vi "Autonomous Independent.vi"() -> ()   [LabVIEW 2016]
doc: "This VI is called when autonomous begins, and will automatically be terminated when autonomous ends. You can carry out timed or sensor driven robot movement independently without needing to return to the caller."
uses:
  <vilib>/Rock Robotics/WPI/ThirdParty/CanMotor/TalonSRX/WPI_CANTalonSRX_APIFeedbackSelect.ctl
  <vilib>/Rock Robotics/WPI/ThirdParty/CanMotor/TalonSRX/WPI_CANTalonSRX_Params.ctl
  <vilib>/Rock Robotics/WPI/ThirdParty/CanMotor/TalonSRX/WPI_CANTalonSRX_APIControlMode.ctl
  <vilib>/Rock Robotics/WPI/Utilities/WPI_GetSetVariantRefNum.vi
  <vilib>/Rock Robotics/Network Tables/NT Read String.vi
  <vilib>/Rock Robotics/Network Tables/NT Write Numeric Array.vi
  <vilib>/Rock Robotics/WPI/RobotDrive/WPI_RobotDriveArcadeDrive_Standard(NoSaturation).vi
  Robot Global Data.vi
panel:
  out "PLAY 2":dbl
  out "PLAY 1":dbl
  in  "stop":bool
  out "Distance":dbl
  out "Current":dbl
  out "CURRENT":dbl
  out "Distance 5":dbl
  out "Distance 4":dbl
  out "Distance 3":dbl
  out "RIGHT SIDE":dbl
  out "Encoder Position 4":dbl
  out "Encoder Position 3":dbl
  out "Encoder Position":dbl
  out "Encoder Position 2":dbl
  # "Be sure to right-click and choose Data Operations>>Make Current Value default if you want to save the array values with the VI"
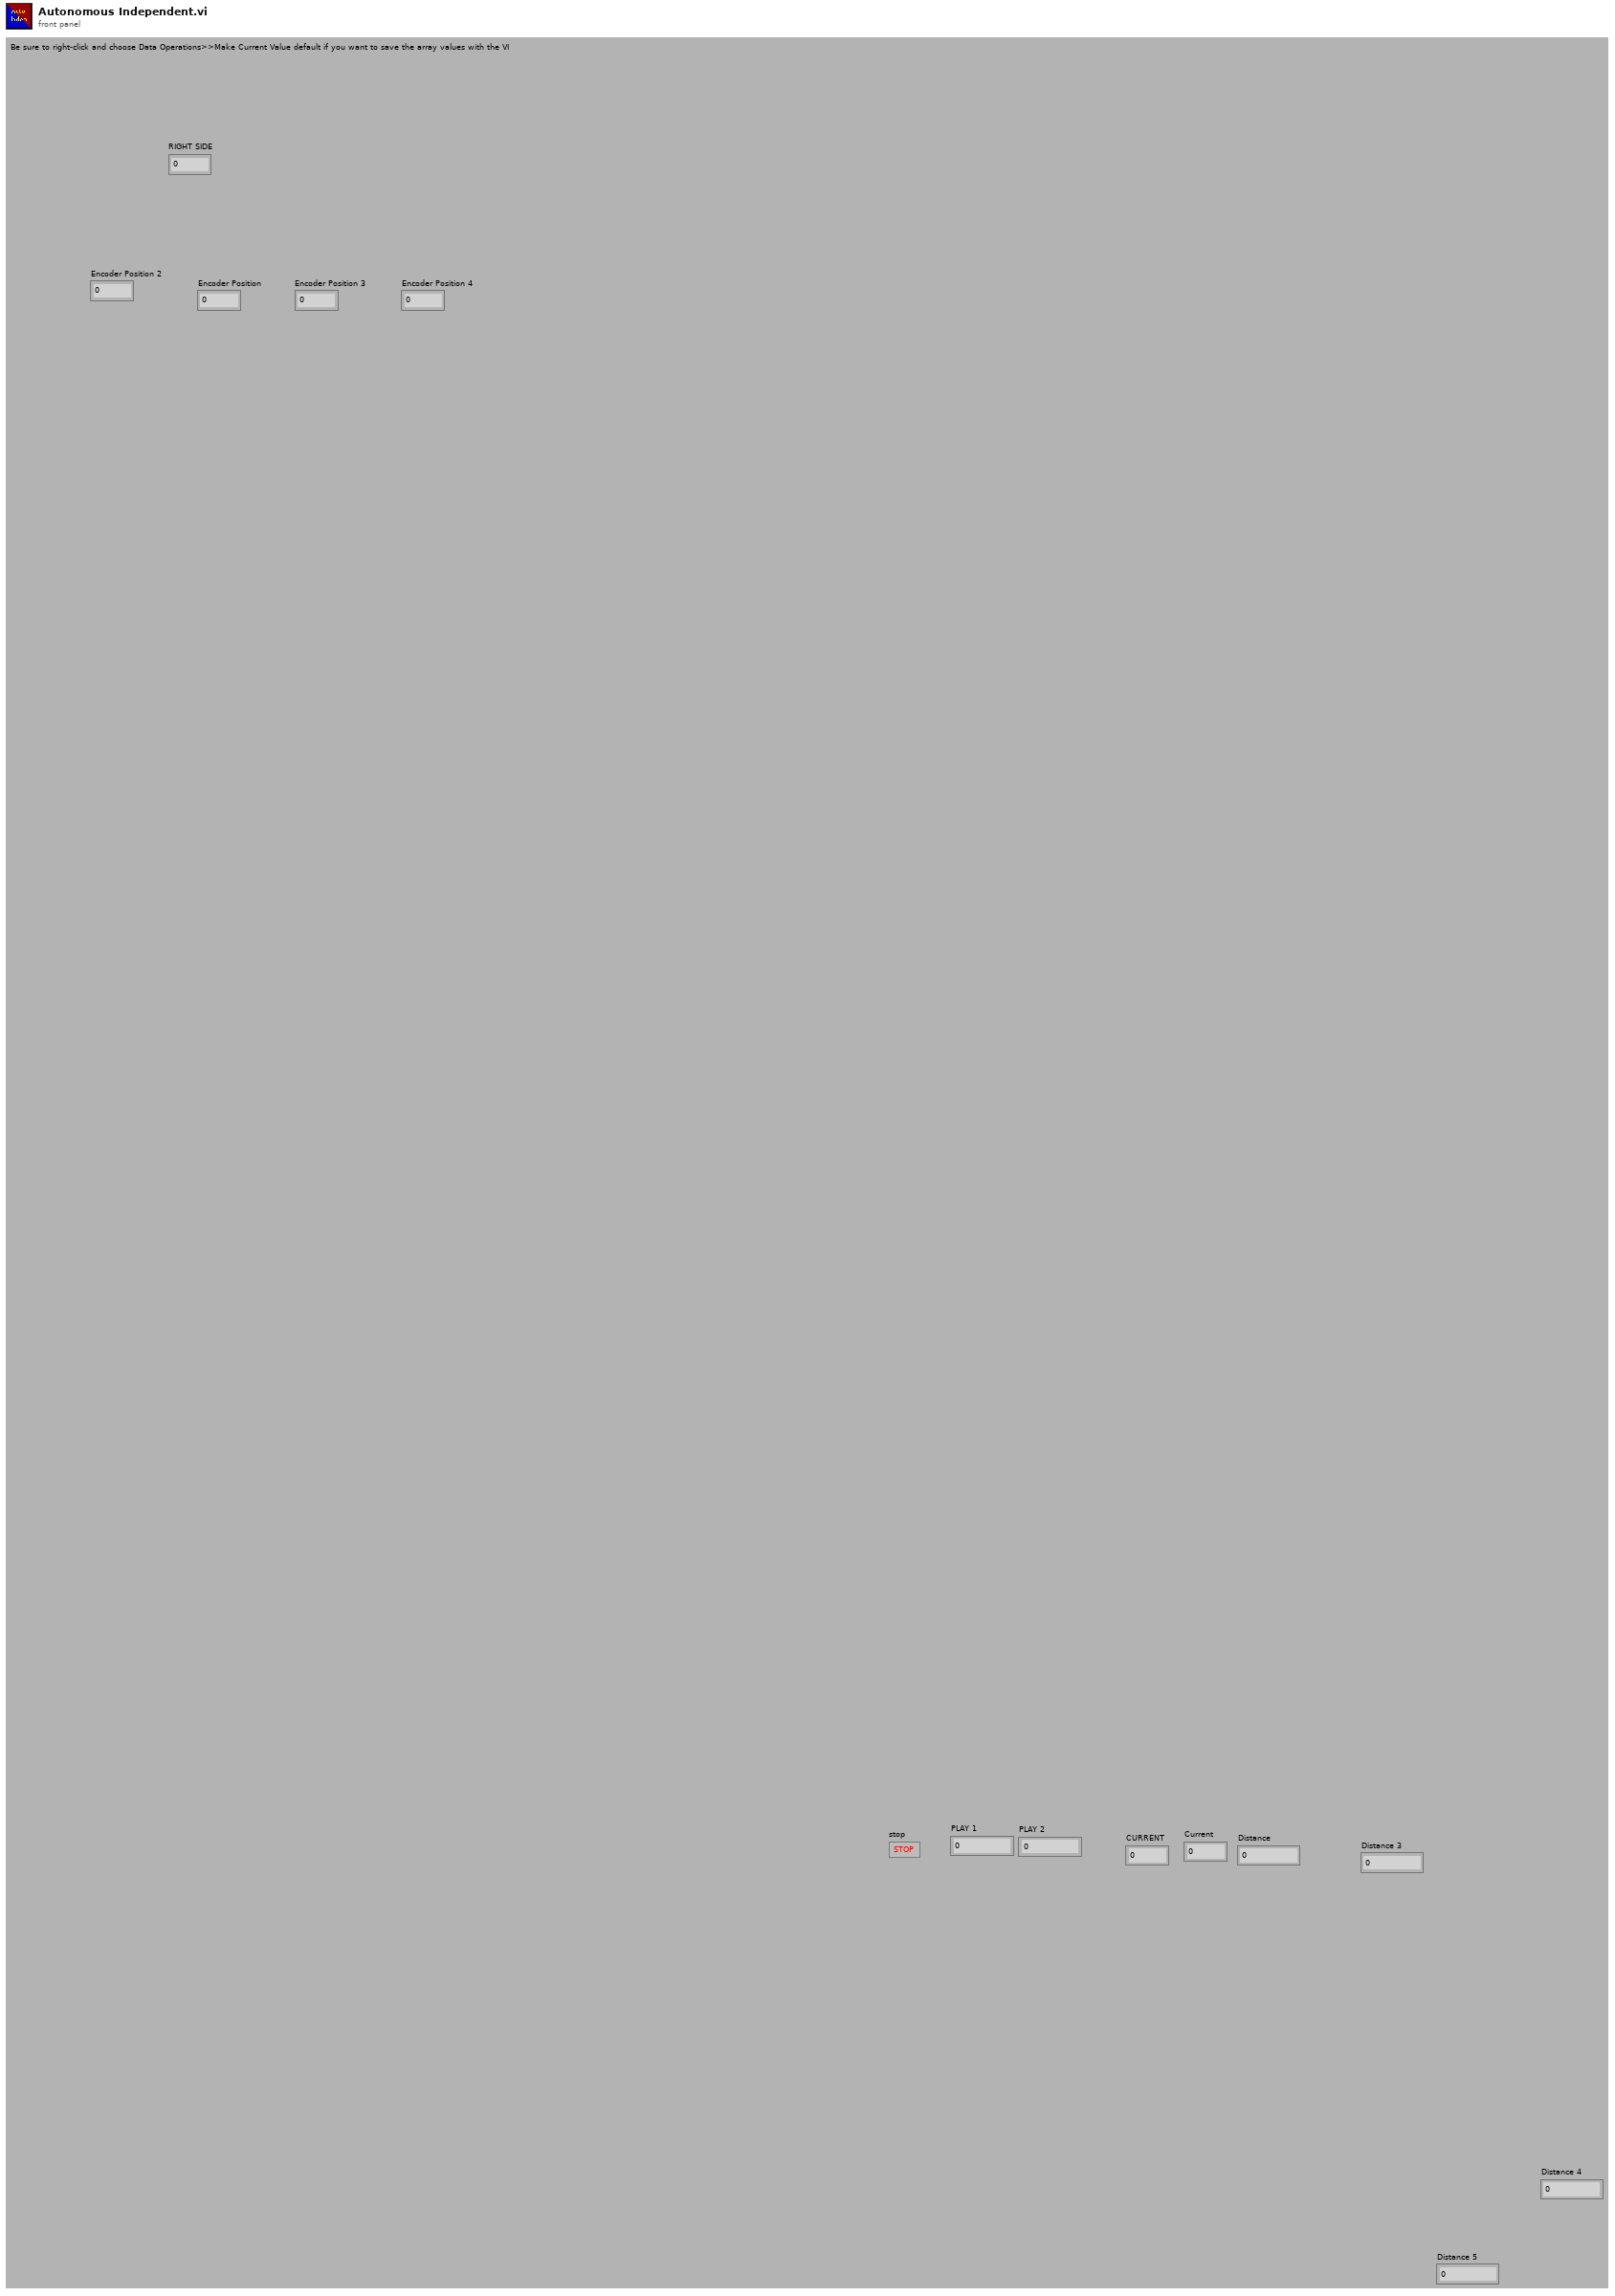
[diagram p1: front panel]
types:
  T1 = typedef "WPI_JoystickDevRef.ctl" = cluster{"Device":T2}
  T2 = typedef "WPI_JoystickDeviceEnum.ctl" = enum16{"USB 0", "USB 1", "USB 2", "USB 3", "USB 4", "USB 5"}
  T3 = typedef "WPI_EncoderDevRef.ctl" = cluster{"DevStatus":errorcluster, "EncoderIndex":T4, "CounterIndex":T5, "DistancePerCount":dbl, "Decoding Type":T6}
  T4 = typedef "FPGA_EncoderIdx.ctl" = enum8{"Enc 0", "Enc 1", "Enc 2", "Enc 3", "Enc 4", "Enc 5", "Enc 6", "Enc 7", "Invalid"}
  T5 = typedef "FPGA_CounterCtrSystemIndex.ctl" = enum8{"Ctr 0", "Ctr 1", "Ctr 2", "Ctr 3", "Ctr 4", "Ctr 5", "Ctr 6", "Ctr 7", "Invalid"}
  T6 = typedef "WPI_EncoderType.ctl" = enum16{"1x", "2x", "4x"}
  T7 = typedef "WPI_MotorControlDeviceRef.ctl" = cluster{"DeviceStatus":errorcluster, "Type":T8, "PWM":cluster{"PWM Channel":T9, "DeadBand":T10}, "CAN":cluster{"Device Number":u8, "SetOutput VI Ref":variant, "GetOutput VI Ref":variant, "Enable VI Ref":variant, "Disable VI Ref":variant, "Data":variant}, "Invert":bool}
  T8 = typedef "WPI_MotorControlType.ctl" = enum16{"PWM", "CAN"}
  T9 = typedef "FPGA_DIOPWMChannel.ctl" = enum8{"PWM 0", "PWM 1", "PWM 2", "PWM 3", "PWM 4", "PWM 5", "PWM 6", "PWM 7", "PWM 8", "PWM 9", "PWM MXP 0", "PWM MXP 1", "PWM MXP 2", "PWM MXP 3", "PWM MXP 4", "PWM MXP 5", "PWM MXP 6", "PWM MXP 7", "PWM MXP 8", "PWM MXP 9", "Invalid"}
  T10 = typedef "WPI_PWMDeadband.ctl" = cluster{"Name":string, "maxPositivePwm":i32, "minPositivePwm":i32, "centerPwm":i32, "maxNegativePwm":i32, "minNegativePwm":i32, "angularRange":u16}
  T11 = typedef "WPI_RobotDriveDevRef.ctl" = cluster{"DevStatus":errorcluster, "Motors[]":T7[], "Square Inputs":bool, "Max Output":dbl}
  T12 = typedef "WPI_CANTalonSRX_APIFeedbackSelect.ctl" = enum16{"Digital Quadrature Encoder", "Analog Potentiometer", "Analog Encoder", "Count on Quad-A (Rising-Edge)", "Count on Quad-A (Falling-Edge)", "CTR Magnetic Enc (Absolute)", "CTR Magnetic Enc (Relative)", "Pulse Width"}
  T13 = typedef "WPI_CANTalonSRX_APIControlMode.ctl" = enum8{"Percent VBus", "Speed", "Position", "Slave", "Unchanged / Invalid", "Voltage Compensation", "Current", "Motion Profile", "Motion Magic"}
  T14 = typedef "WPI_CANTalonSRX_Params.ctl" = u8
  T15 = typedef "WPI_CANTalonSRX_GlobalStatus.ctl" = cluster{"Applied Throttle":dbl, "Module Enabled":bool, "CAN Error":errorcluster, "Closed Loop Error":dbl, "Forward Limit Switch Closed":bool, "Reverse Limit Switch Closed":bool, "Sensor Position":dbl, "Sensor Velocity":dbl, "Current":dbl, "Sticky Fault - Over Temp":bool, "Sticky Fault - Under Voltage":bool, "Sticky Fault - Forward Limit":bool, "Sticky Fault - Reverse Limit":bool, "Sticky Fault - Forward Soft Limit":bool, "Sticky Fault - Reverse Soft Limit":bool, "Brake is Enabled":bool, "Encoder Position":dbl, "Encoder Velocity":dbl, "Encoder Index Count":dbl, "Encoder A Pin State":bool, "Encoder B Pin State":bool, "Encoder Index Pin State":bool, "Analog In":dbl, "Analog In Velocity":dbl, "Temperature (C)":dbl, "Battery Voltage":dbl, "Control 5 Is Supported":bool, "Current Profile Slot Select":dbl, "Pos Div 8":bool, "Vel Div 4":bool, "Pulse Width Position":i32, "Pulse Width Velocity":i32, "Pulse Width Rise To Rise (us)":i32, "Pulse Width Rise To Fall (us)":i32, "Mot Prof Active Is Under Run":bool, "Mot Prof Active Has Under Run":bool, "Mot Prof Active Is Last":bool, "Mot Prof Active Velocity Only":bool, "Mot Prof Active Is Valid":bool, "Mot Prof Buffer Is Full":bool, "Mot Prof Active Profile Slot Select":i32, "Mot Prof NextID":i32, "Mot Prof Count":i32, "Mot Prof Active Velocity":dbl, "Mot Prof Active Position":dbl, "Mot Prof Output Enable":i32, "UsageFrame":u32}
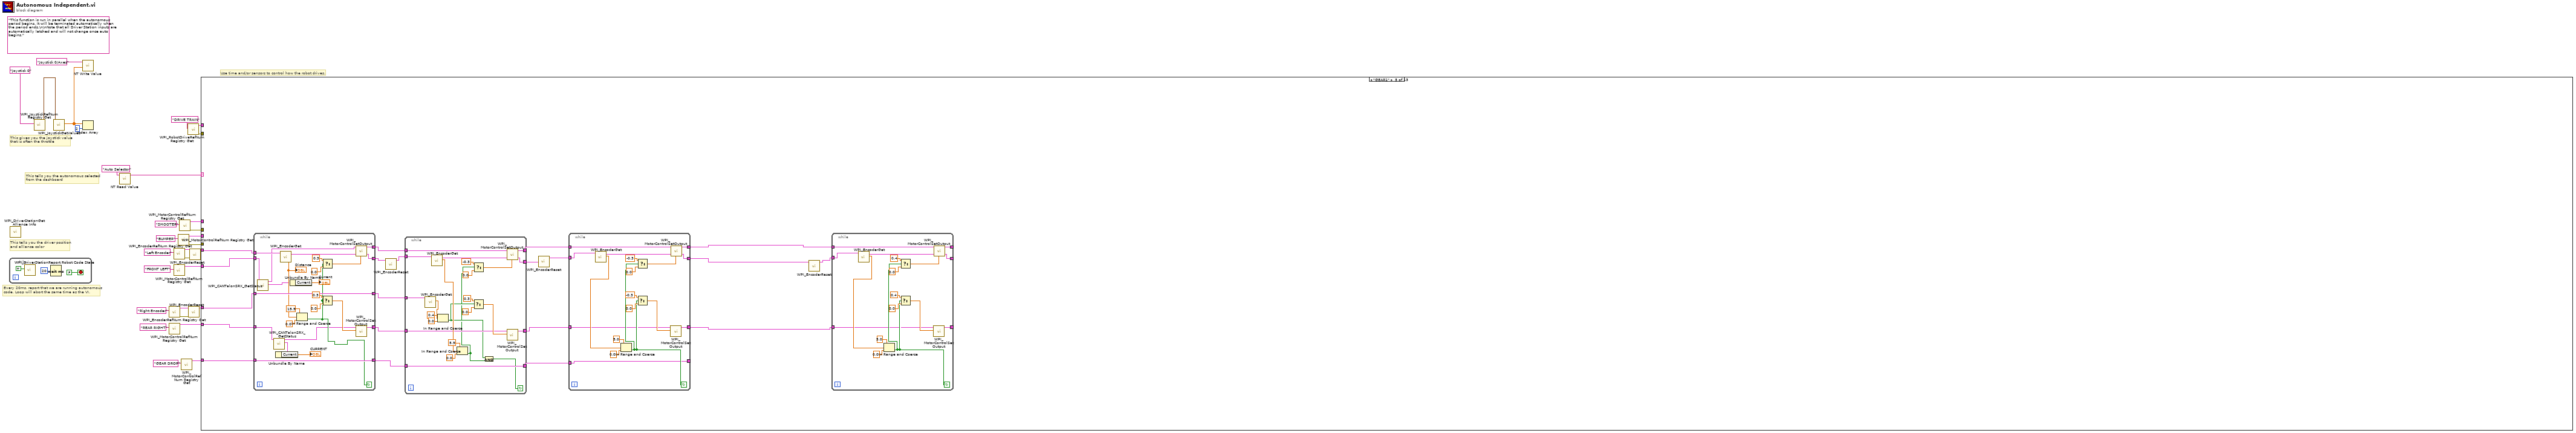
[diagram p0: block diagram]
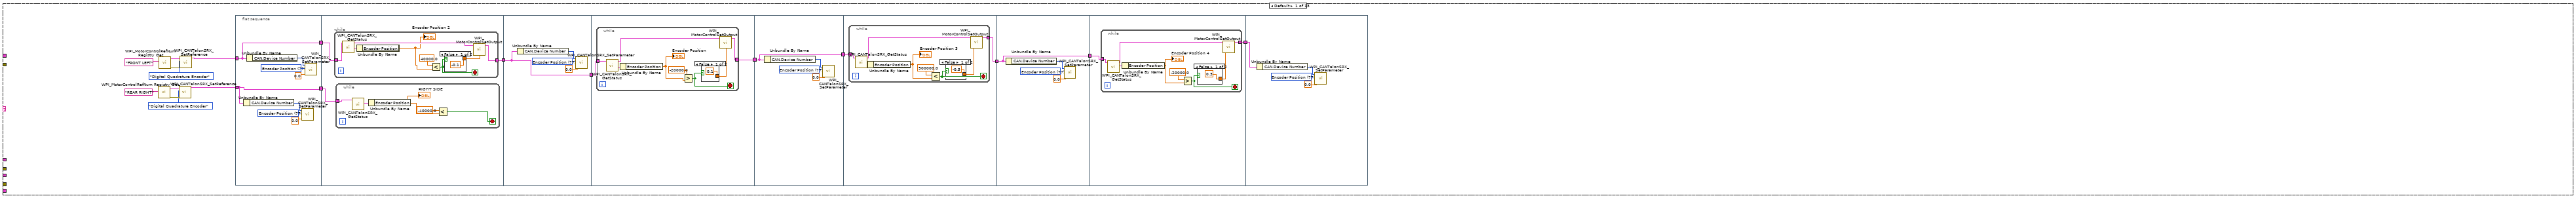
[diagram p2: hidden frame]
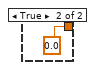
[diagram p3: hidden frame]
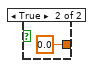
[diagram p4: hidden frame]
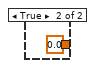
[diagram p5: hidden frame]
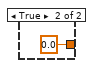
[diagram p6: hidden frame]
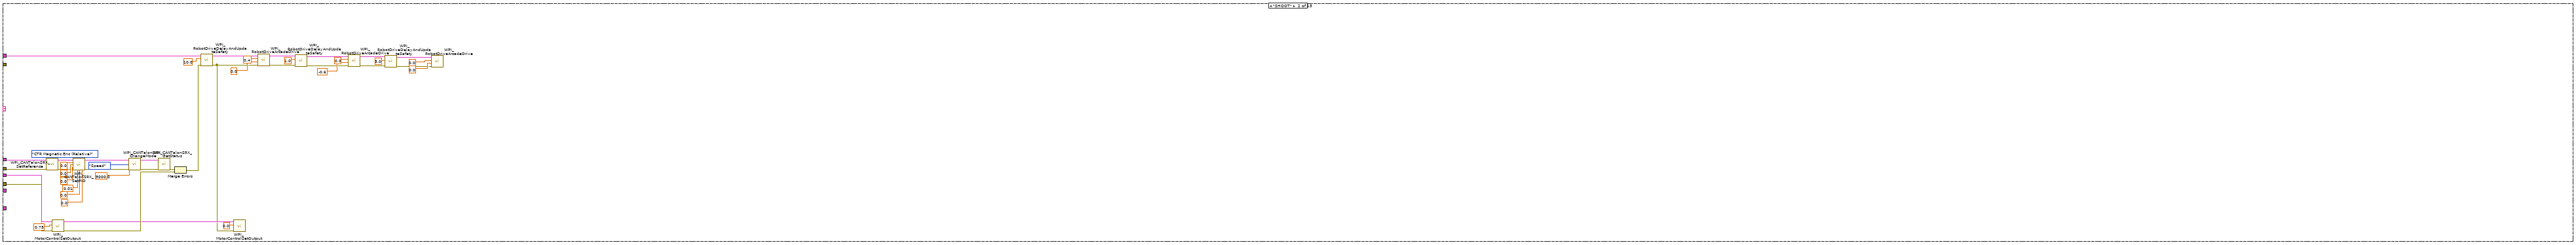
[diagram p7: hidden frame]
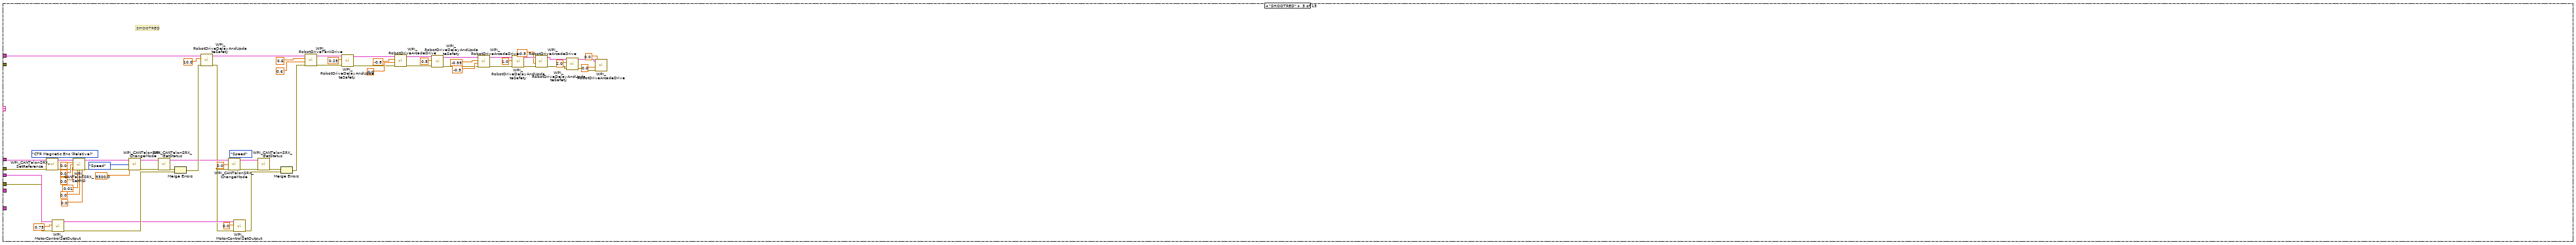
[diagram p8: hidden frame]
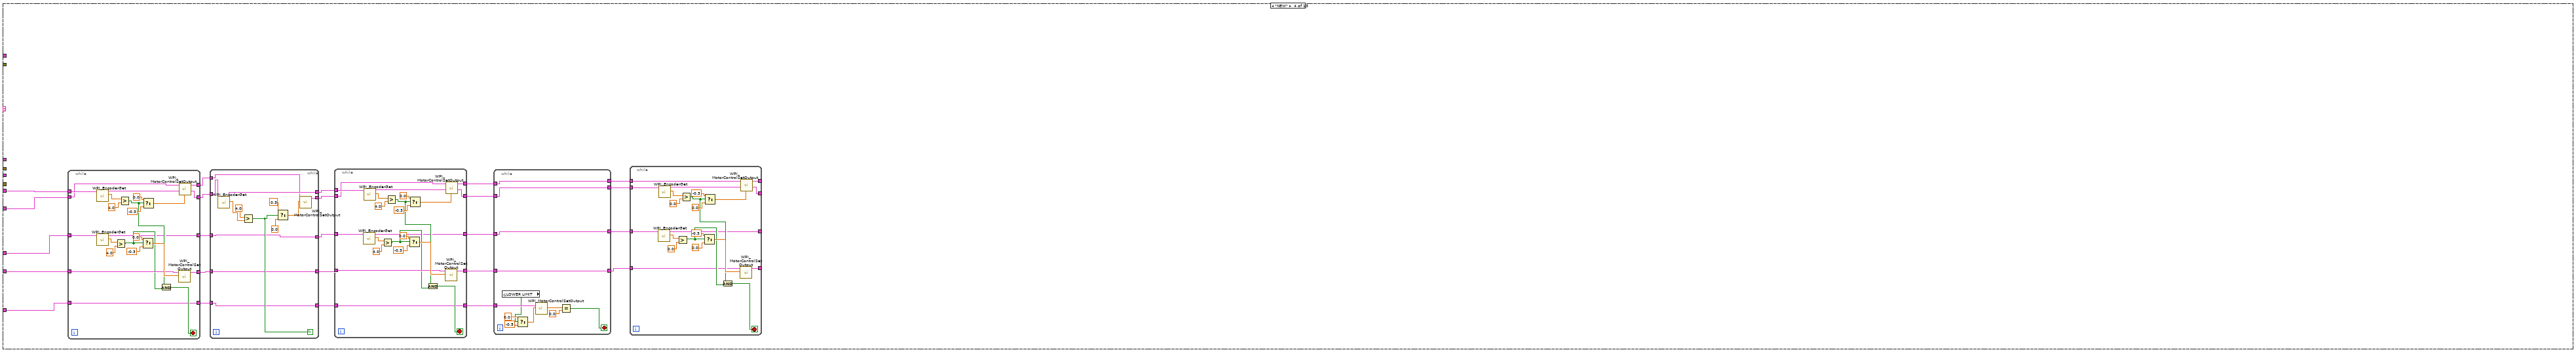
[diagram p9: hidden frame]
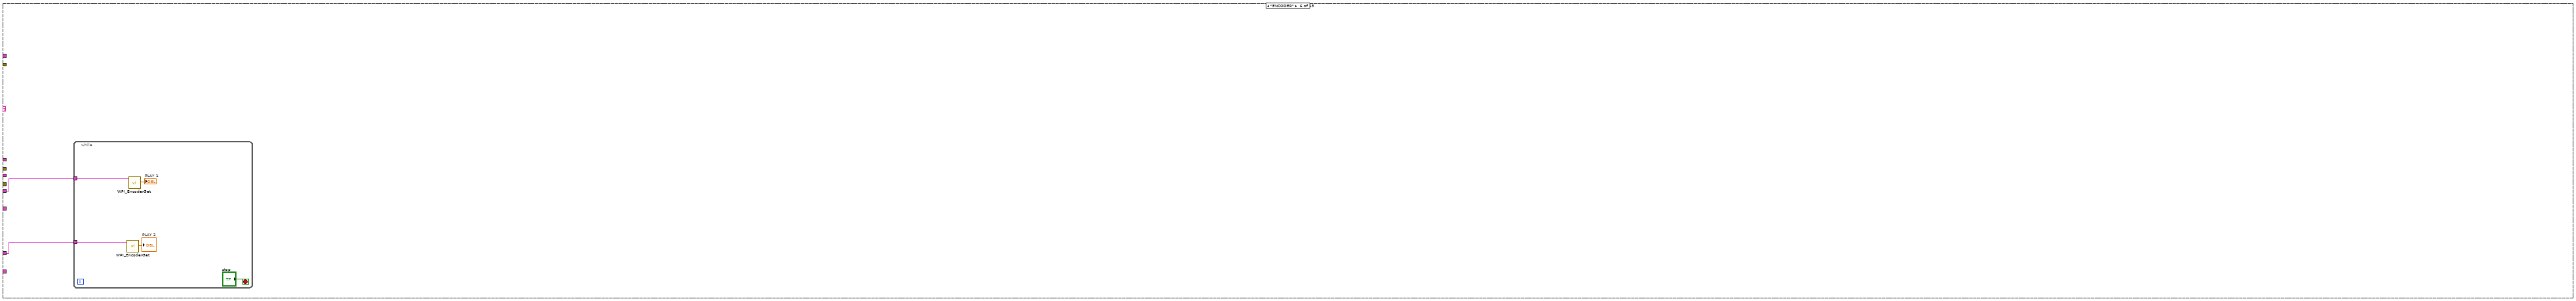
[diagram p10: hidden frame]
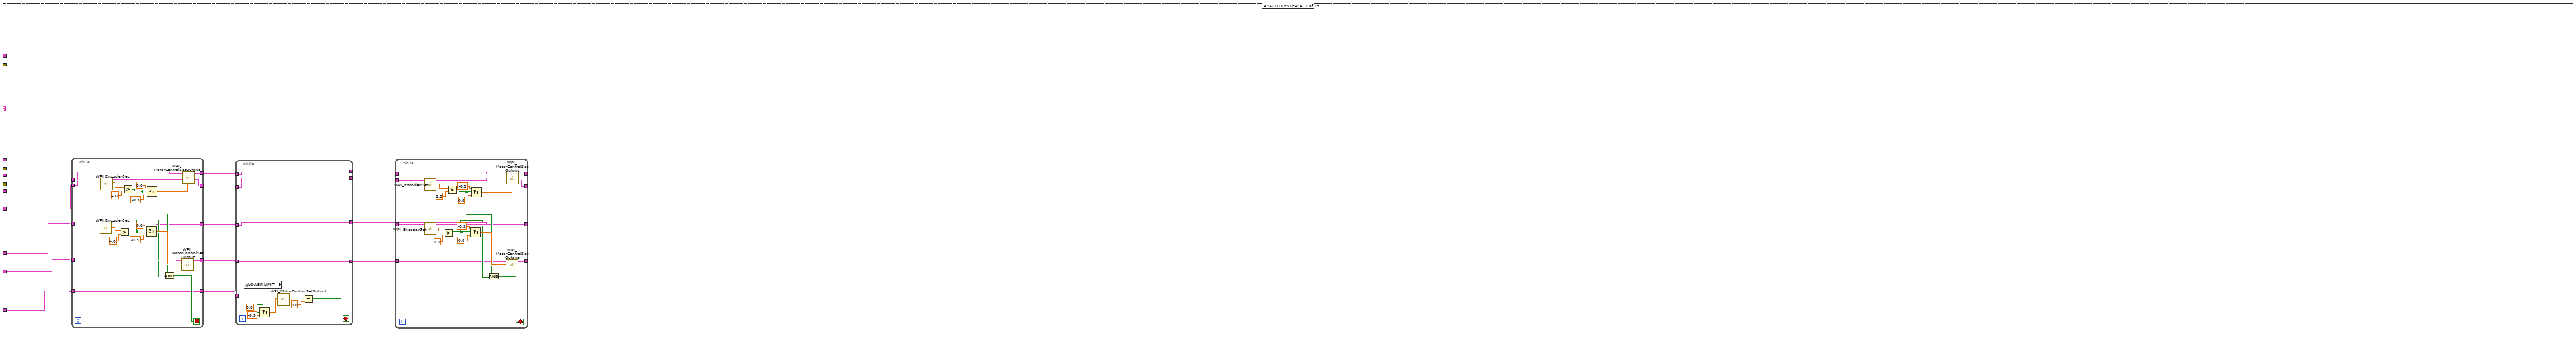
[diagram p11: hidden frame]
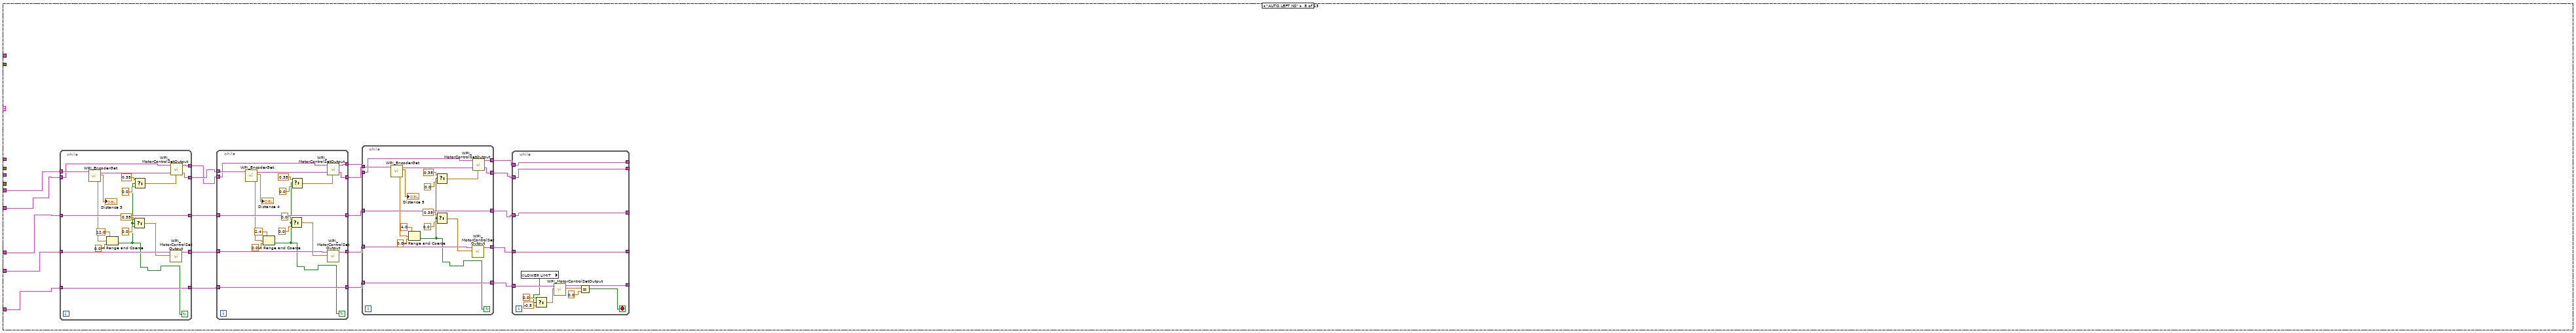
[diagram p12: hidden frame]
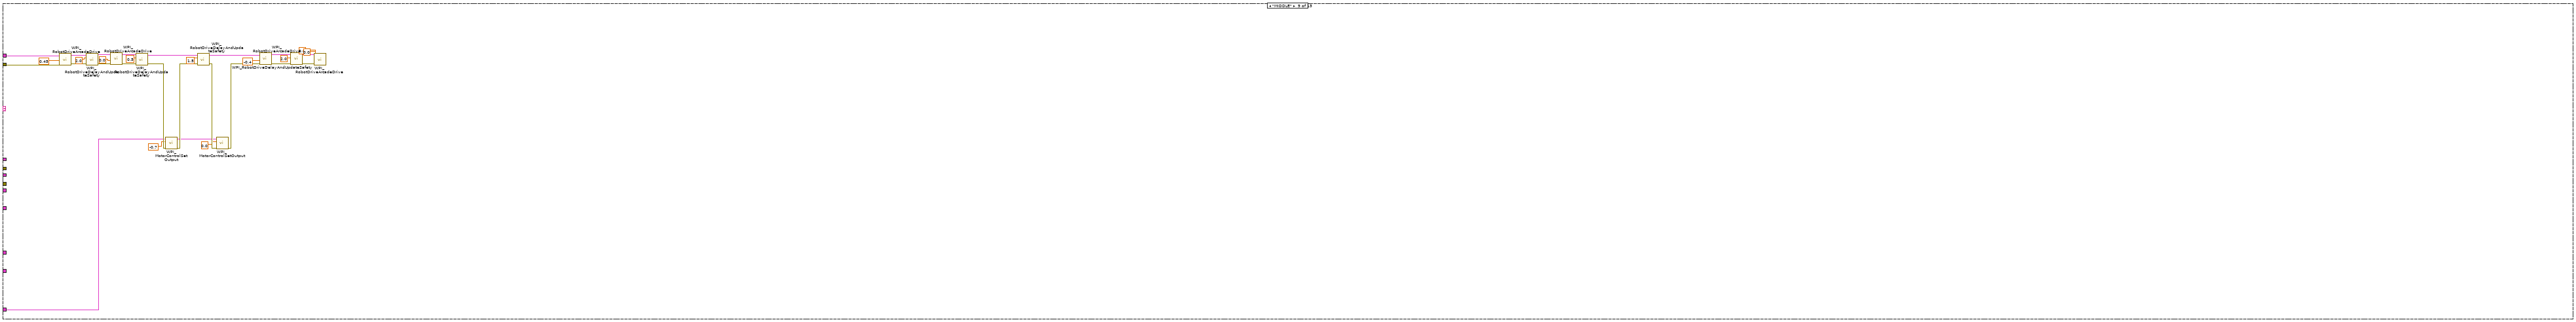
[diagram p13: hidden frame]
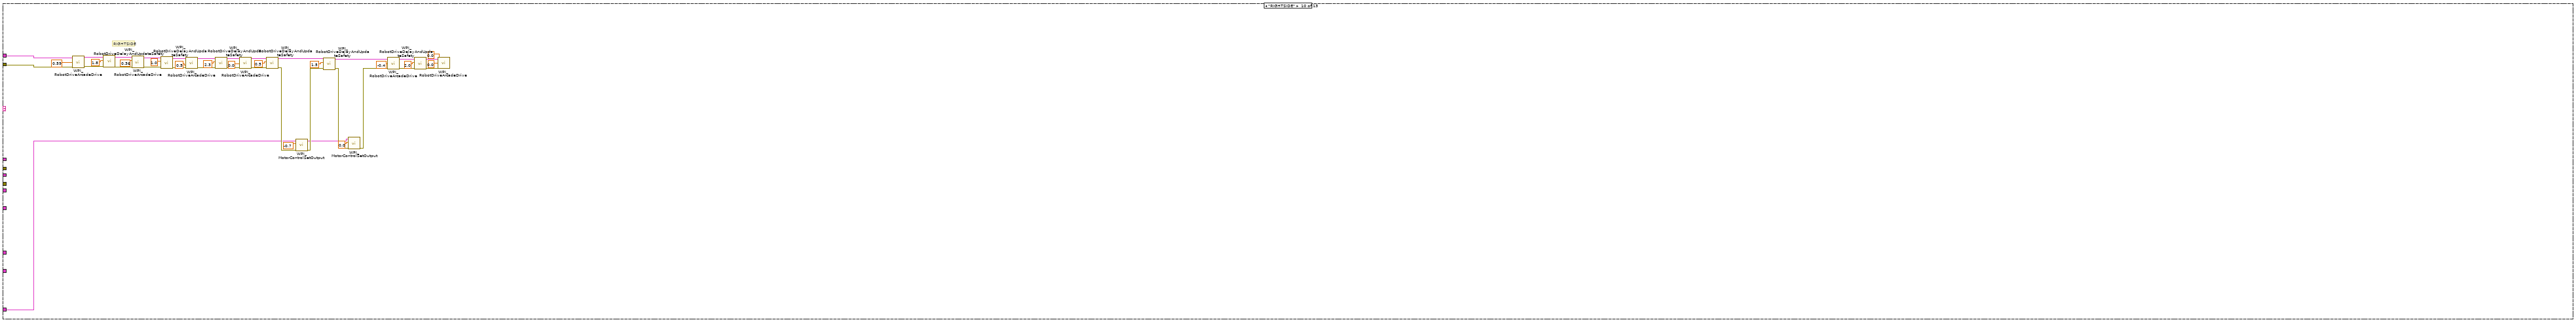
[diagram p14: hidden frame]
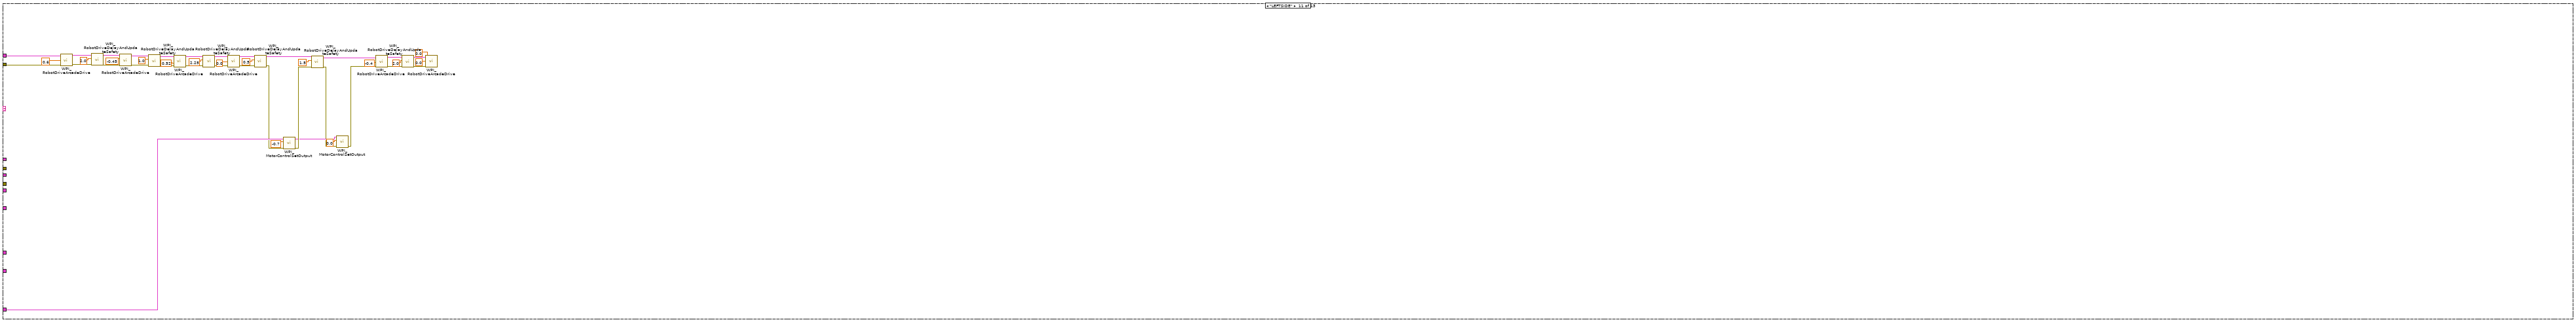
[diagram p15: hidden frame]
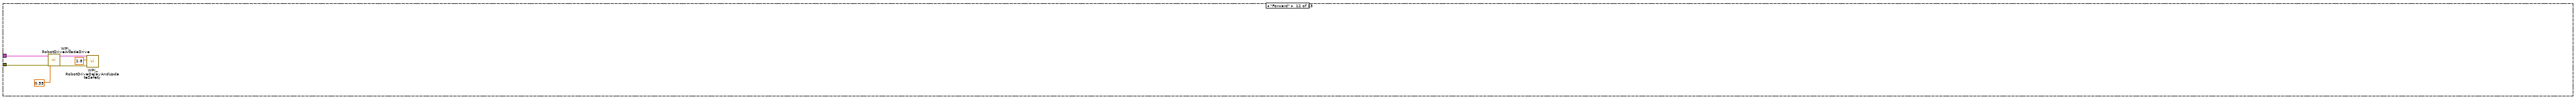
[diagram p16: hidden frame]
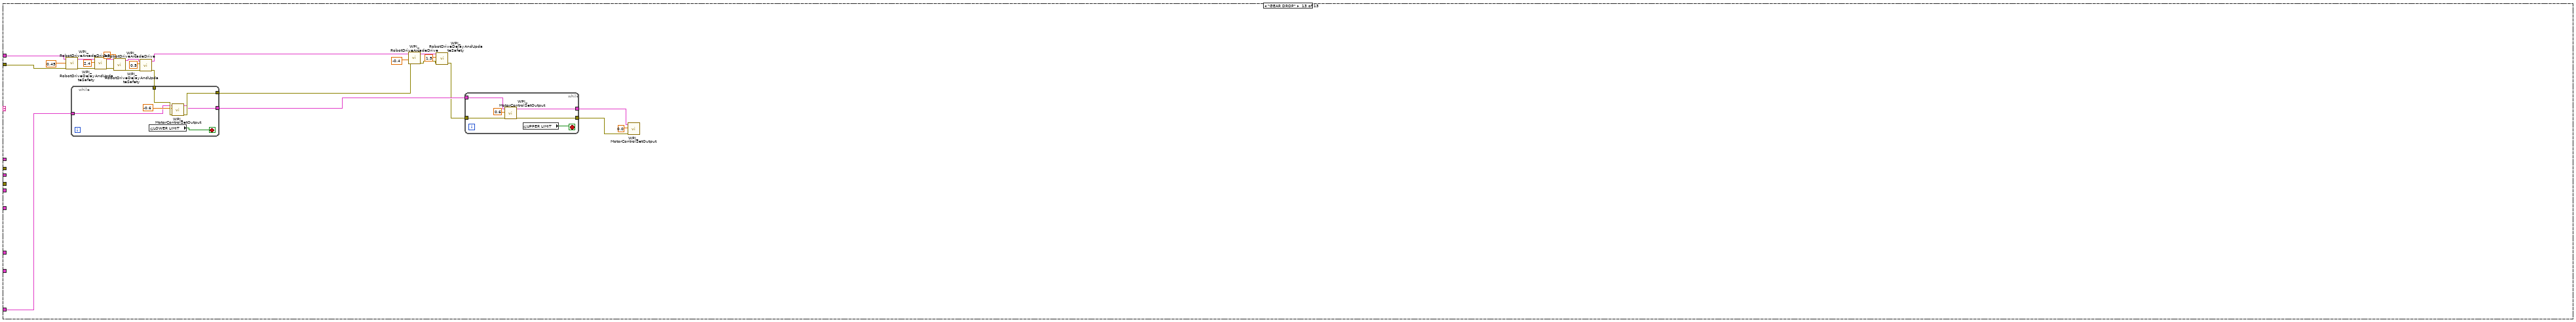
[diagram p17: hidden frame]
diagram:
  (unwired) "This function is run in parallel when the autonomous period begins. It will be terminated automatically when the period ends.\n\nNote that all Driver Station inputs are automatically latched and will not change once auto begins."
  # "Use time and/or sensors to control how the robot drives."
  # "This tells you the autonomous selected\nfrom the dashboard"
  # "Every 20ms, report that we are running autonomous\ncode. Loop will abort the same time as the VI."
  # "This gives you the joystick value\nthat is often the throttle"
  # "This tells you the driver position\nand alliance color"
  n1 = while {
    stop <- FALSE stop-if-true
    n2 = call <vilib>:"WPI_DriverStationReport Robot Code State.vi"("Autonomous"=TRUE) -> ()  [unwired: 10 in, 1 out]
    n3 = Wait (ms)(milliseconds to wait=u32 20) -> ()  [unwired: 1 out]
  }
  n4 = call <vilib>:"WPI_DriverStationGet Alliance Info.vi"() -> ()  [unwired: 12 out]
  n5 = call <vilib>:"WPI_JoystickRefNum Registry Get.vi"("refnum name"="Joystick 0") -> ("JoystickDevRef"=w29:T1)  [unwired: 1 in, 9 out]
  n6 = call <vilib>:"WPI_JoystickGetValues.vi"("JoystickDevRef"=w29) -> ("Axes"=w25:dbl[])  [unwired: 6 in, 4 out]
  n7 = call-poly <vilib>:"NT Write Value.vi"("Numeric Array"=w25, "Name"="Joystick 0/Axes") -> ()  [unwired: 9 in, 1 out]
  n8 = Index Array(array=w25, index=2) -> ()  [unwired: 1 out]
  n9 = call-poly <vilib>:"NT Read Value.vi"("Name"="Auto Selector") -> ("String"=w26:string)  [unwired: 9 in, 1 out]
  n10 = call <vilib>:"WPI_EncoderRefNum Registry Get.vi"("refnum name"="Right Encoder") -> ("error out"=w6:errorcluster, "EncoderDevRef"=w5:T3)  [unwired: 9 in]
  n11 = call <vilib>:"WPI_MotorControlRefNum Registry Get.vi"("refnum name"="REAR RIGHT") -> ("MotorControlDevRef"=w7:T7)  [unwired: 9 in, 1 out]
  n12 = call <vilib>:"WPI_EncoderRefNum Registry Get.vi"("refnum name"="Left Encoder") -> ("error out"=w3:errorcluster, "EncoderDevRef"=w2:T3)  [unwired: 9 in]
  n13 = call <vilib>:"WPI_MotorControlRefNum Registry Get.vi"("refnum name"="FRONT LEFT") -> ("MotorControlDevRef"=w10:T7)  [unwired: 9 in, 1 out]
  n14 = call <vilib>:"WPI_MotorControlRefNum Registry Get.vi"("refnum name"="BUMPER") -> ("error out"=w14:errorcluster, "MotorControlDevRef"=w15:T7)  [unwired: 9 in]
  n15 = call <vilib>:"WPI_MotorControlRefNum Registry Get.vi"("refnum name"="SHOOTER") -> ("error out"=w16:errorcluster, "MotorControlDevRef"=w17:T7)  [unwired: 9 in]
  n16 = call <vilib>:"WPI_MotorControlRefNum Registry Get.vi"("refnum name"="GEAR DROP") -> ("MotorControlDevRef"=w19:T7)  [unwired: 9 in, 1 out]
  n17 = call <vilib>:"WPI_RobotDriveRefNum Registry Get.vi"("refnum name"="DRIVE TRAIN") -> ("error out"=w21:errorcluster, "RobotDriveDevRef"=w22:T11)  [unwired: 9 in]
  n18 = call <vilib>:"WPI_EncoderReset.vi"("error in (no error)"=w6, "EncoderDevRef"=w5) -> ("EncoderDevRef"=w4:T3)  [unwired: 8 in, 1 out]
  n19 = call <vilib>:"WPI_EncoderReset.vi"("error in (no error)"=w3, "EncoderDevRef"=w2) -> ("EncoderDevRef"=w1:T3)  [unwired: 8 in, 1 out]
  n20 = case shown="\"GEAR1\"" w26 {
    tunnel: w22 -> [_ w157 w223 _ _ _ _ _ w649 w652 w735 w741 w766]
    tunnel: w21 -> [_ _ _ _ _ _ _ _ w648 w651 w734 w740 w765]
    tunnel: w19 -> [_ _ _ w249 w371 _ w472 w547 w636 w650 w711 _ w746]
    tunnel: w17 -> [_ w163 w229 _ _ _ _ _ _ _ _ _ _]
    tunnel: w16 -> [_ w162 w228 _ _ _ _ _ _ _ _ _ _]
    tunnel: w15 -> [_ w148 w216 _ _ _ _ _ _ _ _ _ _]
    tunnel: w14 -> [_ w147 w215 _ _ _ _ _ _ _ _ _ _]
    tunnel: w1 -> [_ _ _ w263 w374 w456 w476 w551 _ _ _ _ _]
    tunnel: w10 -> [_ _ _ w262 w375 _ w475 w550 _ _ _ _ _]
    tunnel: w7 -> [_ _ _ w260 w372 _ w473 w548 _ _ _ _ _]
    tunnel: w4 -> [_ _ _ w261 w373 w457 w474 w549 _ _ _ _ _]
    frame Default {
      n21 = call <vilib>:"WPI_MotorControlRefNum Registry Get.vi"("refnum name"="REAR RIGHT") -> ("error out"=w38:errorcluster, "MotorControlDevRef"=w37:T7)  [unwired: 9 in]
      n22 = call <vilib>:"WPI_MotorControlRefNum Registry Get.vi"("refnum name"="FRONT LEFT") -> ("error out"=w50:errorcluster, "MotorControlDevRef"=w51:T7)  [unwired: 9 in]
      n23 = call <vilib>:"WPI_CANTalonSRX_SetReference.vi"("error in (no error)"=w38, "Feedback Reference"=WPI_CANTalonSRX_APIFeedbackSelect."Digital Quadrature Encoder", "CAN Talon SRX Ref"=w37) -> ("CAN Talon SRX Ref"=w35:T7)  [unwired: 7 in, 1 out]
      n24 = call <vilib>:"WPI_CANTalonSRX_SetReference.vi"("error in (no error)"=w50, "Feedback Reference"=WPI_CANTalonSRX_APIFeedbackSelect."Digital Quadrature Encoder", "CAN Talon SRX Ref"=w51) -> ("CAN Talon SRX Ref"=w46:T7)  [unwired: 7 in, 1 out]
      n25 = flat-sequence {
        tunnel: w46 -> [w57]
        tunnel: [w57] -> w45
        tunnel: w35 -> [w53]
        tunnel: [w53] -> w34
        tunnel: [w62] -> w48
        tunnel: w45 -> [w63]
        tunnel: w34 -> [w61]
        tunnel: w48 -> [w79]
        tunnel: [w79] -> w47
        tunnel: w47 -> [w84]
        tunnel: [w83] -> w44
        tunnel: w44 -> [w95]
        tunnel: [w95] -> w43
        tunnel: w43 -> [w100]
        tunnel: [w99] -> w42
        tunnel: w42 -> [w111]
        tunnel: [w111] -> w41
        tunnel: w41 -> [w116]
        tunnel: [w115] -> w40
        tunnel: w40 -> [w127]
        frame #0 {
          w55 = T14 77 items=["Slot 0 - P"=1, "Slot 0 - I"=2, "Slot 0 - D"=3, "Slot 0 - F"=4, "Slot 0 - I Zone"=5, "Slot 0 - Ramp Rate"=6, "Slot 1 - P"=11, "Slot 1 - I"=12, "Slot 1 - D"=13, "Slot 1 - F"=14, "Slot 1 - I Zone"=15, "Slot 1 - Ramp Rate"=16, "Soft Limit - Forward"=21, "Soft Limit - Reverse"=22, "Soft Limit - Forward Enable"=23, "Soft Limit - Reverse Enable"=24, "On Boot - Brake Mode"=31, "On Boot - Limit Normally Closed - Forward"=32, "On Boot - Limit Normally Closed - Reverse"=33, "On Boot - Limit Disabled - Forward"=34, "On Boot - Limit Disabled - Reverse"=35, "Fault - Over Temp"=41, "Fault - Under Voltage"=42, "Fault - Forward Limit"=43, "Fault - Reverse Limit"=44, "Fault - Hardware Failure"=45, "Fault - Forward Soft Limit"=46, "Fault - Reverse Soft Limit"=47, "Sticky Fault - Over Temp"=48, "Sticky Fault - Under Voltage"=49, "Sticky Fault - Forward Limit"=50, "Sticky Fault - Reverse Limit"=51, "Sticky Fault - Forward Soft Limit"=52, "Sticky Fault - Reverse Soft Limit"=53, "Applied Throttle"=61, "Closed-Loop Error"=62, "Select Feedback Device"=63, "Reverse Closed-Loop Output"=64, "Mode Select"=65, "Profile Slot Select"=66, "Ramp Throttle"=67, "Reverse Feedback Sensor"=68, "Limit Switch Enabled"=69, "Limit Switch Closed - Forward"=70, "Limit Switch Closed - Reverse"=71, "Sensor Position"=73, "Sensor Velocity"=74, "Current"=75, "Brake is Enabled"=76, "Encoder Position"=77, "Encoder Velocity"=78, "Encoder Index Rise Events"=79, "Encoder A Pin State"=80, "Encoder B Pin State"=81, "Encoder Index Pin State"=82, "Analog In with Overflow"=83, "Analog In Velocity"=84, "Temperature"=85, "Battery Voltage"=86, "Reset Count"=87, "Reset Flags"=88, "Firmware Version"=89, "Settings Changed"=90, "Quad Filter Enable"=91, "Ignore Disable Broadcast"=92, "I Accumulator"=93, "Status 1 Frame Rate Ms"=94, "Status 2 Frame Rate Ms"=95, "Status 3 Frame Rate Ms"=96, "Status 4 Frame Rate Ms"=97, "Status 6 Frame Rate Ms"=98, "Status 7 Frame Rate Ms"=99, "Enable Index Pin Clear Position"=100, "Peak Positive Output"=104, "Nominal Positive Output"=105, "Peak Negative Output"=106, "Nominal Negative Output"=107, "Quad Index Pin Polarity"=108, "Status 8 Frame Rate Ms"=109, "Allow Position Overflow"=110, "Slot 0 - Allowable Closed-Loop Error"=111, "Number Potentiometer Turns"=112, "Encoder Codes Per Rev"=113, "Pulse Width Decoded Position"=114, "Analog Position"=115, "Voltage Compensation Rate (V/s)"=116, "Slot 1 - Allowable Closed-Loop Error"=117, "Motion Profile Has Underrun Err"=119, "Reserved 120"=120, "Legacy Control Mode"=121, "Motion Magic Acceleration"=122, "Motion Magic Cruise Velocity"=123, "Status 10 Frame Rate"=124, "Current Limit Threshold"=125, "CustomParam0"=137, "CustomParam1"=138, "PersStorageSaving"=139, "ClearPositionOnLimitF"=144, "ClearPositionOnLimitR"=145, "NominalBatteryVoltage"=146, "SampleVelocityPeriod"=147, "SampleVelocityWindow"=148] ("Parameter")
          w59 = T14 77 items=["Slot 0 - P"=1, "Slot 0 - I"=2, "Slot 0 - D"=3, "Slot 0 - F"=4, "Slot 0 - I Zone"=5, "Slot 0 - Ramp Rate"=6, "Slot 1 - P"=11, "Slot 1 - I"=12, "Slot 1 - D"=13, "Slot 1 - F"=14, "Slot 1 - I Zone"=15, "Slot 1 - Ramp Rate"=16, "Soft Limit - Forward"=21, "Soft Limit - Reverse"=22, "Soft Limit - Forward Enable"=23, "Soft Limit - Reverse Enable"=24, "On Boot - Brake Mode"=31, "On Boot - Limit Normally Closed - Forward"=32, "On Boot - Limit Normally Closed - Reverse"=33, "On Boot - Limit Disabled - Forward"=34, "On Boot - Limit Disabled - Reverse"=35, "Fault - Over Temp"=41, "Fault - Under Voltage"=42, "Fault - Forward Limit"=43, "Fault - Reverse Limit"=44, "Fault - Hardware Failure"=45, "Fault - Forward Soft Limit"=46, "Fault - Reverse Soft Limit"=47, "Sticky Fault - Over Temp"=48, "Sticky Fault - Under Voltage"=49, "Sticky Fault - Forward Limit"=50, "Sticky Fault - Reverse Limit"=51, "Sticky Fault - Forward Soft Limit"=52, "Sticky Fault - Reverse Soft Limit"=53, "Applied Throttle"=61, "Closed-Loop Error"=62, "Select Feedback Device"=63, "Reverse Closed-Loop Output"=64, "Mode Select"=65, "Profile Slot Select"=66, "Ramp Throttle"=67, "Reverse Feedback Sensor"=68, "Limit Switch Enabled"=69, "Limit Switch Closed - Forward"=70, "Limit Switch Closed - Reverse"=71, "Sensor Position"=73, "Sensor Velocity"=74, "Current"=75, "Brake is Enabled"=76, "Encoder Position"=77, "Encoder Velocity"=78, "Encoder Index Rise Events"=79, "Encoder A Pin State"=80, "Encoder B Pin State"=81, "Encoder Index Pin State"=82, "Analog In with Overflow"=83, "Analog In Velocity"=84, "Temperature"=85, "Battery Voltage"=86, "Reset Count"=87, "Reset Flags"=88, "Firmware Version"=89, "Settings Changed"=90, "Quad Filter Enable"=91, "Ignore Disable Broadcast"=92, "I Accumulator"=93, "Status 1 Frame Rate Ms"=94, "Status 2 Frame Rate Ms"=95, "Status 3 Frame Rate Ms"=96, "Status 4 Frame Rate Ms"=97, "Status 6 Frame Rate Ms"=98, "Status 7 Frame Rate Ms"=99, "Enable Index Pin Clear Position"=100, "Peak Positive Output"=104, "Nominal Positive Output"=105, "Peak Negative Output"=106, "Nominal Negative Output"=107, "Quad Index Pin Polarity"=108, "Status 8 Frame Rate Ms"=109, "Allow Position Overflow"=110, "Slot 0 - Allowable Closed-Loop Error"=111, "Number Potentiometer Turns"=112, "Encoder Codes Per Rev"=113, "Pulse Width Decoded Position"=114, "Analog Position"=115, "Voltage Compensation Rate (V/s)"=116, "Slot 1 - Allowable Closed-Loop Error"=117, "Motion Profile Has Underrun Err"=119, "Reserved 120"=120, "Legacy Control Mode"=121, "Motion Magic Acceleration"=122, "Motion Magic Cruise Velocity"=123, "Status 10 Frame Rate"=124, "Current Limit Threshold"=125, "CustomParam0"=137, "CustomParam1"=138, "PersStorageSaving"=139, "ClearPositionOnLimitF"=144, "ClearPositionOnLimitR"=145, "NominalBatteryVoltage"=146, "SampleVelocityPeriod"=147, "SampleVelocityWindow"=148] ("Parameter")
          n26 = Unbundle By Name(w53) -> ("CAN.Device Number"=w54:u8)
          n27 = Unbundle By Name(w57) -> ("CAN.Device Number"=w60:u8)
          n28 = call <vilib>:"WPI_CANTalonSRX_SetParameter.vi"("Value"=0.0, "Parameter"=w55, "Device ID (0)"=w54) -> ()  [unwired: 7 in, 2 out]
          n29 = call <vilib>:"WPI_CANTalonSRX_SetParameter.vi"("Value"=0.0, "Parameter"=w59, "Device ID (0)"=w60) -> ()  [unwired: 7 in, 2 out]
        }
        frame #1 {
          n30 = while {
            tunnel: w63 -> [w70]
            tunnel: [w69] -> w62
            stop <- w73 stop-if-true
            n31 = call <vilib>:"WPI_CANTalonSRX_GetStatus.vi"("CAN Talon SRX Ref"=w70) -> ("Talon SRX Status"=w76:T15, "CAN Talon SRX Ref"=w75:T7)  [unwired: 8 in, 1 out]
            n32 = Unbundle By Name(w76) -> ("Encoder Position"=w72:dbl)
            "Encoder Position 2" <- w72
            n33 = Less?(x=40000.0, y=w72) -> (x < y?=w73:bool)
            n34 = case shown="False" w73 {
              tunnel: [-0.1 ("x") 0.0 ("x")] -> w74
              frame False {
              }
              frame True {
              }
            }
            n35 = call <vilib>:"WPI_MotorControlSetOutput.vi"("Output"=w74, "MotorControlDevRef"=w75) -> ("MotorControlDevRef"=w69:T7)  [unwired: 7 in, 2 out]
          }
          n36 = while {
            tunnel: w61 -> [w68]
            stop <- w65 stop-if-true
            n37 = call <vilib>:"WPI_CANTalonSRX_GetStatus.vi"("CAN Talon SRX Ref"=w68) -> ("Talon SRX Status"=w64:T15)  [unwired: 8 in, 2 out]
            n38 = Unbundle By Name(w64) -> ("Encoder Position"=w67:dbl)
            "RIGHT SIDE" <- w67
            n39 = Less?(x=-40000.0, y=w67) -> (x < y?=w65:bool)
          }
        }
        frame #2 {
          w81 = T14 77 items=["Slot 0 - P"=1, "Slot 0 - I"=2, "Slot 0 - D"=3, "Slot 0 - F"=4, "Slot 0 - I Zone"=5, "Slot 0 - Ramp Rate"=6, "Slot 1 - P"=11, "Slot 1 - I"=12, "Slot 1 - D"=13, "Slot 1 - F"=14, "Slot 1 - I Zone"=15, "Slot 1 - Ramp Rate"=16, "Soft Limit - Forward"=21, "Soft Limit - Reverse"=22, "Soft Limit - Forward Enable"=23, "Soft Limit - Reverse Enable"=24, "On Boot - Brake Mode"=31, "On Boot - Limit Normally Closed - Forward"=32, "On Boot - Limit Normally Closed - Reverse"=33, "On Boot - Limit Disabled - Forward"=34, "On Boot - Limit Disabled - Reverse"=35, "Fault - Over Temp"=41, "Fault - Under Voltage"=42, "Fault - Forward Limit"=43, "Fault - Reverse Limit"=44, "Fault - Hardware Failure"=45, "Fault - Forward Soft Limit"=46, "Fault - Reverse Soft Limit"=47, "Sticky Fault - Over Temp"=48, "Sticky Fault - Under Voltage"=49, "Sticky Fault - Forward Limit"=50, "Sticky Fault - Reverse Limit"=51, "Sticky Fault - Forward Soft Limit"=52, "Sticky Fault - Reverse Soft Limit"=53, "Applied Throttle"=61, "Closed-Loop Error"=62, "Select Feedback Device"=63, "Reverse Closed-Loop Output"=64, "Mode Select"=65, "Profile Slot Select"=66, "Ramp Throttle"=67, "Reverse Feedback Sensor"=68, "Limit Switch Enabled"=69, "Limit Switch Closed - Forward"=70, "Limit Switch Closed - Reverse"=71, "Sensor Position"=73, "Sensor Velocity"=74, "Current"=75, "Brake is Enabled"=76, "Encoder Position"=77, "Encoder Velocity"=78, "Encoder Index Rise Events"=79, "Encoder A Pin State"=80, "Encoder B Pin State"=81, "Encoder Index Pin State"=82, "Analog In with Overflow"=83, "Analog In Velocity"=84, "Temperature"=85, "Battery Voltage"=86, "Reset Count"=87, "Reset Flags"=88, "Firmware Version"=89, "Settings Changed"=90, "Quad Filter Enable"=91, "Ignore Disable Broadcast"=92, "I Accumulator"=93, "Status 1 Frame Rate Ms"=94, "Status 2 Frame Rate Ms"=95, "Status 3 Frame Rate Ms"=96, "Status 4 Frame Rate Ms"=97, "Status 6 Frame Rate Ms"=98, "Status 7 Frame Rate Ms"=99, "Enable Index Pin Clear Position"=100, "Peak Positive Output"=104, "Nominal Positive Output"=105, "Peak Negative Output"=106, "Nominal Negative Output"=107, "Quad Index Pin Polarity"=108, "Status 8 Frame Rate Ms"=109, "Allow Position Overflow"=110, "Slot 0 - Allowable Closed-Loop Error"=111, "Number Potentiometer Turns"=112, "Encoder Codes Per Rev"=113, "Pulse Width Decoded Position"=114, "Analog Position"=115, "Voltage Compensation Rate (V/s)"=116, "Slot 1 - Allowable Closed-Loop Error"=117, "Motion Profile Has Underrun Err"=119, "Reserved 120"=120, "Legacy Control Mode"=121, "Motion Magic Acceleration"=122, "Motion Magic Cruise Velocity"=123, "Status 10 Frame Rate"=124, "Current Limit Threshold"=125, "CustomParam0"=137, "CustomParam1"=138, "PersStorageSaving"=139, "ClearPositionOnLimitF"=144, "ClearPositionOnLimitR"=145, "NominalBatteryVoltage"=146, "SampleVelocityPeriod"=147, "SampleVelocityWindow"=148] ("Parameter")
          n40 = Unbundle By Name(w79) -> ("CAN.Device Number"=w82:u8)
          n41 = call <vilib>:"WPI_CANTalonSRX_SetParameter.vi"("Value"=0.0, "Parameter"=w81, "Device ID (0)"=w82) -> ()  [unwired: 7 in, 2 out]
        }
        frame #3 {
          n42 = while {
            tunnel: w84 -> [w86]
            tunnel: [w85] -> w83
            stop <- w89 stop-if-true
            n43 = call <vilib>:"WPI_CANTalonSRX_GetStatus.vi"("CAN Talon SRX Ref"=w86) -> ("Talon SRX Status"=w92:T15, "CAN Talon SRX Ref"=w91:T7)  [unwired: 8 in, 1 out]
            n44 = Unbundle By Name(w92) -> ("Encoder Position"=w88:dbl)
            "Encoder Position" <- w88
            n45 = Greater?(x=-20000.0 ("y"), y=w88) -> (0:w89:bool)
            n46 = case shown="False" w89 {
              tunnel: [0.1 ("x") 0.0 ("x")] -> w90
              frame False {
              }
              frame True {
              }
            }
            n47 = call <vilib>:"WPI_MotorControlSetOutput.vi"("Output"=w90, "MotorControlDevRef"=w91) -> ("MotorControlDevRef"=w85:T7)  [unwired: 7 in, 2 out]
          }
        }
        frame #4 {
          w97 = T14 77 items=["Slot 0 - P"=1, "Slot 0 - I"=2, "Slot 0 - D"=3, "Slot 0 - F"=4, "Slot 0 - I Zone"=5, "Slot 0 - Ramp Rate"=6, "Slot 1 - P"=11, "Slot 1 - I"=12, "Slot 1 - D"=13, "Slot 1 - F"=14, "Slot 1 - I Zone"=15, "Slot 1 - Ramp Rate"=16, "Soft Limit - Forward"=21, "Soft Limit - Reverse"=22, "Soft Limit - Forward Enable"=23, "Soft Limit - Reverse Enable"=24, "On Boot - Brake Mode"=31, "On Boot - Limit Normally Closed - Forward"=32, "On Boot - Limit Normally Closed - Reverse"=33, "On Boot - Limit Disabled - Forward"=34, "On Boot - Limit Disabled - Reverse"=35, "Fault - Over Temp"=41, "Fault - Under Voltage"=42, "Fault - Forward Limit"=43, "Fault - Reverse Limit"=44, "Fault - Hardware Failure"=45, "Fault - Forward Soft Limit"=46, "Fault - Reverse Soft Limit"=47, "Sticky Fault - Over Temp"=48, "Sticky Fault - Under Voltage"=49, "Sticky Fault - Forward Limit"=50, "Sticky Fault - Reverse Limit"=51, "Sticky Fault - Forward Soft Limit"=52, "Sticky Fault - Reverse Soft Limit"=53, "Applied Throttle"=61, "Closed-Loop Error"=62, "Select Feedback Device"=63, "Reverse Closed-Loop Output"=64, "Mode Select"=65, "Profile Slot Select"=66, "Ramp Throttle"=67, "Reverse Feedback Sensor"=68, "Limit Switch Enabled"=69, "Limit Switch Closed - Forward"=70, "Limit Switch Closed - Reverse"=71, "Sensor Position"=73, "Sensor Velocity"=74, "Current"=75, "Brake is Enabled"=76, "Encoder Position"=77, "Encoder Velocity"=78, "Encoder Index Rise Events"=79, "Encoder A Pin State"=80, "Encoder B Pin State"=81, "Encoder Index Pin State"=82, "Analog In with Overflow"=83, "Analog In Velocity"=84, "Temperature"=85, "Battery Voltage"=86, "Reset Count"=87, "Reset Flags"=88, "Firmware Version"=89, "Settings Changed"=90, "Quad Filter Enable"=91, "Ignore Disable Broadcast"=92, "I Accumulator"=93, "Status 1 Frame Rate Ms"=94, "Status 2 Frame Rate Ms"=95, "Status 3 Frame Rate Ms"=96, "Status 4 Frame Rate Ms"=97, "Status 6 Frame Rate Ms"=98, "Status 7 Frame Rate Ms"=99, "Enable Index Pin Clear Position"=100, "Peak Positive Output"=104, "Nominal Positive Output"=105, "Peak Negative Output"=106, "Nominal Negative Output"=107, "Quad Index Pin Polarity"=108, "Status 8 Frame Rate Ms"=109, "Allow Position Overflow"=110, "Slot 0 - Allowable Closed-Loop Error"=111, "Number Potentiometer Turns"=112, "Encoder Codes Per Rev"=113, "Pulse Width Decoded Position"=114, "Analog Position"=115, "Voltage Compensation Rate (V/s)"=116, "Slot 1 - Allowable Closed-Loop Error"=117, "Motion Profile Has Underrun Err"=119, "Reserved 120"=120, "Legacy Control Mode"=121, "Motion Magic Acceleration"=122, "Motion Magic Cruise Velocity"=123, "Status 10 Frame Rate"=124, "Current Limit Threshold"=125, "CustomParam0"=137, "CustomParam1"=138, "PersStorageSaving"=139, "ClearPositionOnLimitF"=144, "ClearPositionOnLimitR"=145, "NominalBatteryVoltage"=146, "SampleVelocityPeriod"=147, "SampleVelocityWindow"=148] ("Parameter")
          n48 = Unbundle By Name(w95) -> ("CAN.Device Number"=w98:u8)
          n49 = call <vilib>:"WPI_CANTalonSRX_SetParameter.vi"("Value"=0.0, "Parameter"=w97, "Device ID (0)"=w98) -> ()  [unwired: 7 in, 2 out]
        }
        frame #5 {
          n50 = while {
            tunnel: w100 -> [w102]
            tunnel: [w101] -> w99
            stop <- w105 stop-if-true
            n51 = call <vilib>:"WPI_CANTalonSRX_GetStatus.vi"("CAN Talon SRX Ref"=w102) -> ("Talon SRX Status"=w108:T15, "CAN Talon SRX Ref"=w107:T7)  [unwired: 8 in, 1 out]
            n52 = Unbundle By Name(w108) -> ("Encoder Position"=w104:dbl)
            "Encoder Position 3" <- w104
            n53 = Less?(x=500000.0, y=w104) -> (x < y?=w105:bool)
            n54 = case shown="False" w105 {
              tunnel: [-0.5 ("x") 0.0 ("x")] -> w106
              frame False {
              }
              frame True {
              }
            }
            n55 = call <vilib>:"WPI_MotorControlSetOutput.vi"("Output"=w106, "MotorControlDevRef"=w107) -> ("MotorControlDevRef"=w101:T7)  [unwired: 7 in, 2 out]
          }
        }
        frame #6 {
          w113 = T14 77 items=["Slot 0 - P"=1, "Slot 0 - I"=2, "Slot 0 - D"=3, "Slot 0 - F"=4, "Slot 0 - I Zone"=5, "Slot 0 - Ramp Rate"=6, "Slot 1 - P"=11, "Slot 1 - I"=12, "Slot 1 - D"=13, "Slot 1 - F"=14, "Slot 1 - I Zone"=15, "Slot 1 - Ramp Rate"=16, "Soft Limit - Forward"=21, "Soft Limit - Reverse"=22, "Soft Limit - Forward Enable"=23, "Soft Limit - Reverse Enable"=24, "On Boot - Brake Mode"=31, "On Boot - Limit Normally Closed - Forward"=32, "On Boot - Limit Normally Closed - Reverse"=33, "On Boot - Limit Disabled - Forward"=34, "On Boot - Limit Disabled - Reverse"=35, "Fault - Over Temp"=41, "Fault - Under Voltage"=42, "Fault - Forward Limit"=43, "Fault - Reverse Limit"=44, "Fault - Hardware Failure"=45, "Fault - Forward Soft Limit"=46, "Fault - Reverse Soft Limit"=47, "Sticky Fault - Over Temp"=48, "Sticky Fault - Under Voltage"=49, "Sticky Fault - Forward Limit"=50, "Sticky Fault - Reverse Limit"=51, "Sticky Fault - Forward Soft Limit"=52, "Sticky Fault - Reverse Soft Limit"=53, "Applied Throttle"=61, "Closed-Loop Error"=62, "Select Feedback Device"=63, "Reverse Closed-Loop Output"=64, "Mode Select"=65, "Profile Slot Select"=66, "Ramp Throttle"=67, "Reverse Feedback Sensor"=68, "Limit Switch Enabled"=69, "Limit Switch Closed - Forward"=70, "Limit Switch Closed - Reverse"=71, "Sensor Position"=73, "Sensor Velocity"=74, "Current"=75, "Brake is Enabled"=76, "Encoder Position"=77, "Encoder Velocity"=78, "Encoder Index Rise Events"=79, "Encoder A Pin State"=80, "Encoder B Pin State"=81, "Encoder Index Pin State"=82, "Analog In with Overflow"=83, "Analog In Velocity"=84, "Temperature"=85, "Battery Voltage"=86, "Reset Count"=87, "Reset Flags"=88, "Firmware Version"=89, "Settings Changed"=90, "Quad Filter Enable"=91, "Ignore Disable Broadcast"=92, "I Accumulator"=93, "Status 1 Frame Rate Ms"=94, "Status 2 Frame Rate Ms"=95, "Status 3 Frame Rate Ms"=96, "Status 4 Frame Rate Ms"=97, "Status 6 Frame Rate Ms"=98, "Status 7 Frame Rate Ms"=99, "Enable Index Pin Clear Position"=100, "Peak Positive Output"=104, "Nominal Positive Output"=105, "Peak Negative Output"=106, "Nominal Negative Output"=107, "Quad Index Pin Polarity"=108, "Status 8 Frame Rate Ms"=109, "Allow Position Overflow"=110, "Slot 0 - Allowable Closed-Loop Error"=111, "Number Potentiometer Turns"=112, "Encoder Codes Per Rev"=113, "Pulse Width Decoded Position"=114, "Analog Position"=115, "Voltage Compensation Rate (V/s)"=116, "Slot 1 - Allowable Closed-Loop Error"=117, "Motion Profile Has Underrun Err"=119, "Reserved 120"=120, "Legacy Control Mode"=121, "Motion Magic Acceleration"=122, "Motion Magic Cruise Velocity"=123, "Status 10 Frame Rate"=124, "Current Limit Threshold"=125, "CustomParam0"=137, "CustomParam1"=138, "PersStorageSaving"=139, "ClearPositionOnLimitF"=144, "ClearPositionOnLimitR"=145, "NominalBatteryVoltage"=146, "SampleVelocityPeriod"=147, "SampleVelocityWindow"=148] ("Parameter")
          n56 = Unbundle By Name(w111) -> ("CAN.Device Number"=w112:u8)
          n57 = call <vilib>:"WPI_CANTalonSRX_SetParameter.vi"("Value"=0.0, "Parameter"=w113, "Device ID (0)"=w112) -> ()  [unwired: 7 in, 2 out]
        }
        frame #7 {
          n58 = while {
            tunnel: w116 -> [w118]
            tunnel: [w117] -> w115
            stop <- w121 stop-if-true
            n59 = call <vilib>:"WPI_CANTalonSRX_GetStatus.vi"("CAN Talon SRX Ref"=w118) -> ("Talon SRX Status"=w124:T15, "CAN Talon SRX Ref"=w123:T7)  [unwired: 8 in, 1 out]
            n60 = Unbundle By Name(w124) -> ("Encoder Position"=w120:dbl)
            "Encoder Position 4" <- w120
            n61 = Greater?(x=-20000.0, y=w120) -> (0:w121:bool)
            n62 = case shown="False" w121 {
              tunnel: [0.3 ("x") 0.0 ("x")] -> w122
              frame False {
              }
              frame True {
              }
            }
            n63 = call <vilib>:"WPI_MotorControlSetOutput.vi"("Output"=w122, "MotorControlDevRef"=w123) -> ("MotorControlDevRef"=w117:T7)  [unwired: 7 in, 2 out]
          }
        }
        frame #8 {
          w129 = T14 77 items=["Slot 0 - P"=1, "Slot 0 - I"=2, "Slot 0 - D"=3, "Slot 0 - F"=4, "Slot 0 - I Zone"=5, "Slot 0 - Ramp Rate"=6, "Slot 1 - P"=11, "Slot 1 - I"=12, "Slot 1 - D"=13, "Slot 1 - F"=14, "Slot 1 - I Zone"=15, "Slot 1 - Ramp Rate"=16, "Soft Limit - Forward"=21, "Soft Limit - Reverse"=22, "Soft Limit - Forward Enable"=23, "Soft Limit - Reverse Enable"=24, "On Boot - Brake Mode"=31, "On Boot - Limit Normally Closed - Forward"=32, "On Boot - Limit Normally Closed - Reverse"=33, "On Boot - Limit Disabled - Forward"=34, "On Boot - Limit Disabled - Reverse"=35, "Fault - Over Temp"=41, "Fault - Under Voltage"=42, "Fault - Forward Limit"=43, "Fault - Reverse Limit"=44, "Fault - Hardware Failure"=45, "Fault - Forward Soft Limit"=46, "Fault - Reverse Soft Limit"=47, "Sticky Fault - Over Temp"=48, "Sticky Fault - Under Voltage"=49, "Sticky Fault - Forward Limit"=50, "Sticky Fault - Reverse Limit"=51, "Sticky Fault - Forward Soft Limit"=52, "Sticky Fault - Reverse Soft Limit"=53, "Applied Throttle"=61, "Closed-Loop Error"=62, "Select Feedback Device"=63, "Reverse Closed-Loop Output"=64, "Mode Select"=65, "Profile Slot Select"=66, "Ramp Throttle"=67, "Reverse Feedback Sensor"=68, "Limit Switch Enabled"=69, "Limit Switch Closed - Forward"=70, "Limit Switch Closed - Reverse"=71, "Sensor Position"=73, "Sensor Velocity"=74, "Current"=75, "Brake is Enabled"=76, "Encoder Position"=77, "Encoder Velocity"=78, "Encoder Index Rise Events"=79, "Encoder A Pin State"=80, "Encoder B Pin State"=81, "Encoder Index Pin State"=82, "Analog In with Overflow"=83, "Analog In Velocity"=84, "Temperature"=85, "Battery Voltage"=86, "Reset Count"=87, "Reset Flags"=88, "Firmware Version"=89, "Settings Changed"=90, "Quad Filter Enable"=91, "Ignore Disable Broadcast"=92, "I Accumulator"=93, "Status 1 Frame Rate Ms"=94, "Status 2 Frame Rate Ms"=95, "Status 3 Frame Rate Ms"=96, "Status 4 Frame Rate Ms"=97, "Status 6 Frame Rate Ms"=98, "Status 7 Frame Rate Ms"=99, "Enable Index Pin Clear Position"=100, "Peak Positive Output"=104, "Nominal Positive Output"=105, "Peak Negative Output"=106, "Nominal Negative Output"=107, "Quad Index Pin Polarity"=108, "Status 8 Frame Rate Ms"=109, "Allow Position Overflow"=110, "Slot 0 - Allowable Closed-Loop Error"=111, "Number Potentiometer Turns"=112, "Encoder Codes Per Rev"=113, "Pulse Width Decoded Position"=114, "Analog Position"=115, "Voltage Compensation Rate (V/s)"=116, "Slot 1 - Allowable Closed-Loop Error"=117, "Motion Profile Has Underrun Err"=119, "Reserved 120"=120, "Legacy Control Mode"=121, "Motion Magic Acceleration"=122, "Motion Magic Cruise Velocity"=123, "Status 10 Frame Rate"=124, "Current Limit Threshold"=125, "CustomParam0"=137, "CustomParam1"=138, "PersStorageSaving"=139, "ClearPositionOnLimitF"=144, "ClearPositionOnLimitR"=145, "NominalBatteryVoltage"=146, "SampleVelocityPeriod"=147, "SampleVelocityWindow"=148] ("Parameter")
          n64 = Unbundle By Name(w127) -> ("CAN.Device Number"=w128:u8)
          n65 = call <vilib>:"WPI_CANTalonSRX_SetParameter.vi"("Value"=0.0, "Parameter"=w129, "Device ID (0)"=w128) -> ()  [unwired: 7 in, 2 out]
        }
      }
    }
    frame "SHOOT" {
      n66 = call <vilib>:"WPI_CANTalonSRX_SetReference.vi"("error in (no error)"=w162, "Feedback Reference"=WPI_CANTalonSRX_APIFeedbackSelect."CTR Magnetic Enc (Relative)", "CAN Talon SRX Ref"=w163) -> ("error out"=w161:errorcluster, "CAN Talon SRX Ref"=w171:T7)  [unwired: 7 in]
      n67 = call <vilib>:"WPI_MotorControlSetOutput.vi"("error in (no error)"=w147, "Output"=0.75, "MotorControlDevRef"=w148) -> ("error out"=w144:errorcluster, "MotorControlDevRef"=w142:T7)  [unwired: 6 in, 1 out]
      n68 = call <vilib>:"WPI_CANTalonSRX_SetPID.vi"("CAN Talon SRX Ref"=w171, "P"=0.0, "I"=0.0, "D"=0.0, "error in (no error)"=w161, "F"=0.01, "I Zone"=0.0, "Ramp Rate"=0.0) -> ("CAN Talon SRX Ref"=w168:T7, "error out"=w160:errorcluster)  [unwired: 6 in]
      n69 = call <vilib>:"WPI_CANTalonSRX_ChangeMode.vi"("error in (no error)"=w160, "Output"=9000.0 ("y"), "Control Mode"=WPI_CANTalonSRX_APIControlMode."Speed", "CAN Talon SRX Ref"=w168) -> ("error out"=w159:errorcluster, "CAN Talon SRX Ref"=w164:T7)  [unwired: 6 in]
      n70 = call <vilib>:"WPI_CANTalonSRX_GetStatus.vi"("error in (no error)"=w159, "CAN Talon SRX Ref"=w164) -> ("error out"=w145:errorcluster)  [unwired: 7 in, 2 out]
      n71 = Merge Errors(w145, w144) -> (w143:errorcluster)
      n72 = call <vilib>:"WPI_RobotDriveDelayAndUpdateSafety.vi"("error in (no error)"=w143, "Delay (s)"=10.0, "RobotDriveDevRef"=w157) -> ("error out"=w141:errorcluster, "RobotDriveDevRef 2"=w158:T11)  [unwired: 7 in]
      n73 = call <vilib>:"WPI_MotorControlSetOutput.vi"("error in (no error)"=w141, "Output"=0.0, "MotorControlDevRef"=w142) -> ()  [unwired: 6 in, 3 out]
      n74 = call-poly <vilib>:"WPI_RobotDriveArcadeDrive.vi"("error in (no error)"=w141, "Y axis value"=0.0, "X axis value"=0.4, "RobotDriveDevRef"=w158) -> ("error out"=w154:errorcluster, "RobotDriveDevRef"=w155:T11)  [unwired: 5 in, 1 out]
      n75 = call <vilib>:"WPI_RobotDriveDelayAndUpdateSafety.vi"("error in (no error)"=w154, "Delay (s)"=1.0, "RobotDriveDevRef"=w155) -> ("error out"=w134:errorcluster, "RobotDriveDevRef 2"=w133:T11)  [unwired: 7 in]
      n76 = call-poly <vilib>:"WPI_RobotDriveArcadeDrive.vi"("error in (no error)"=w134, "Y axis value"=-0.6, "X axis value"=0.0, "RobotDriveDevRef"=w133) -> ("error out"=w137:errorcluster, "RobotDriveDevRef"=w138:T11)  [unwired: 5 in, 1 out]
      n77 = call <vilib>:"WPI_RobotDriveDelayAndUpdateSafety.vi"("error in (no error)"=w137, "Delay (s)"=3.0, "RobotDriveDevRef"=w138) -> ("error out"=w131:errorcluster, "RobotDriveDevRef 2"=w132:T11)  [unwired: 7 in]
      n78 = call-poly <vilib>:"WPI_RobotDriveArcadeDrive.vi"("error in (no error)"=w131, "Y axis value"=0.0, "X axis value"=0.0, "RobotDriveDevRef"=w132) -> ()  [unwired: 5 in, 3 out]
    }
    frame "SHOOTRED" {
      # "SHOOTRED"
      n79 = call <vilib>:"WPI_CANTalonSRX_SetReference.vi"("error in (no error)"=w228, "Feedback Reference"=WPI_CANTalonSRX_APIFeedbackSelect."CTR Magnetic Enc (Relative)", "CAN Talon SRX Ref"=w229) -> ("error out"=w227:errorcluster, "CAN Talon SRX Ref"=w237:T7)  [unwired: 7 in]
      n80 = call <vilib>:"WPI_MotorControlSetOutput.vi"("error in (no error)"=w215, "Output"=0.75, "MotorControlDevRef"=w216) -> ("error out"=w212:errorcluster, "MotorControlDevRef"=w210:T7)  [unwired: 6 in, 1 out]
      n81 = call <vilib>:"WPI_CANTalonSRX_SetPID.vi"("CAN Talon SRX Ref"=w237, "P"=0.0, "I"=0.0, "D"=0.0, "error in (no error)"=w227, "F"=0.01, "I Zone"=0.0, "Ramp Rate"=0.0) -> ("CAN Talon SRX Ref"=w234:T7, "error out"=w226:errorcluster)  [unwired: 6 in]
      n82 = call <vilib>:"WPI_CANTalonSRX_ChangeMode.vi"("error in (no error)"=w226, "Output"=9300.0 ("y"), "Control Mode"=WPI_CANTalonSRX_APIControlMode."Speed", "CAN Talon SRX Ref"=w234) -> ("error out"=w225:errorcluster, "CAN Talon SRX Ref"=w230:T7)  [unwired: 6 in]
      n83 = call <vilib>:"WPI_CANTalonSRX_GetStatus.vi"("error in (no error)"=w225, "CAN Talon SRX Ref"=w230) -> ("error out"=w213:errorcluster, "CAN Talon SRX Ref"=w195:T7)  [unwired: 7 in, 1 out]
      n84 = Merge Errors(w213, w212) -> (w211:errorcluster)
      n85 = call <vilib>:"WPI_RobotDriveDelayAndUpdateSafety.vi"("error in (no error)"=w211, "Delay (s)"=10.0, "RobotDriveDevRef"=w223) -> ("error out"=w194:errorcluster, "RobotDriveDevRef 2"=w224:T11)  [unwired: 7 in]
      n86 = call <vilib>:"WPI_CANTalonSRX_ChangeMode.vi"("error in (no error)"=w194, "Output"=0.0 ("y"), "Control Mode"=WPI_CANTalonSRX_APIControlMode."Speed", "CAN Talon SRX Ref"=w195) -> ("error out"=w196:errorcluster, "CAN Talon SRX Ref"=w197:T7)  [unwired: 6 in]
      n87 = call <vilib>:"WPI_MotorControlSetOutput.vi"("error in (no error)"=w194, "Output"=0.0, "MotorControlDevRef"=w210) -> ("error out"=w192:errorcluster)  [unwired: 6 in, 2 out]
      n88 = call <vilib>:"WPI_CANTalonSRX_GetStatus.vi"("error in (no error)"=w196, "CAN Talon SRX Ref"=w197) -> ("error out"=w193:errorcluster)  [unwired: 7 in, 2 out]
      n89 = Merge Errors(w193, w192) -> (w191:errorcluster)
      n90 = call <vilib>:"WPI_RobotDriveTankDrive.vi"("error in (no error)"=w191, "Right axis value"=0.6 ("Y axis value"), "Left axis value"=0.6, "RobotDriveDevRef"=w224) -> ("error out"=w221:errorcluster, "RobotDriveDevRef"=w222:T11)  [unwired: 5 in, 1 out]
      n91 = call <vilib>:"WPI_RobotDriveDelayAndUpdateSafety.vi"("error in (no error)"=w221, "Delay (s)"=0.25, "RobotDriveDevRef"=w222) -> ("error out"=w203:errorcluster, "RobotDriveDevRef 2"=w202:T11)  [unwired: 7 in]
      n92 = call-poly <vilib>:"WPI_RobotDriveArcadeDrive.vi"("error in (no error)"=w203, "Y axis value"=0.0, "X axis value"=-0.8, "RobotDriveDevRef"=w202) -> ("error out"=w206:errorcluster, "RobotDriveDevRef"=w207:T11)  [unwired: 5 in, 1 out]
      n93 = call <vilib>:"WPI_RobotDriveDelayAndUpdateSafety.vi"("error in (no error)"=w206, "Delay (s)"=0.5, "RobotDriveDevRef"=w207) -> ("error out"=w200:errorcluster, "RobotDriveDevRef 2"=w201:T11)  [unwired: 7 in]
      n94 = call-poly <vilib>:"WPI_RobotDriveArcadeDrive.vi"("error in (no error)"=w200, "Y axis value"=-0.5, "X axis value"=-0.55, "RobotDriveDevRef"=w201) -> ("error out"=w189:errorcluster, "RobotDriveDevRef"=w190:T11)  [unwired: 5 in, 1 out]
      n95 = call <vilib>:"WPI_RobotDriveDelayAndUpdateSafety.vi"("error in (no error)"=w189, "Delay (s)"=1.0, "RobotDriveDevRef"=w190) -> ("error out"=w187:errorcluster, "RobotDriveDevRef 2"=w186:T11)  [unwired: 7 in]
      n96 = call-poly <vilib>:"WPI_RobotDriveArcadeDrive.vi"("error in (no error)"=w187, "Y axis value"=-0.5 ("X axis value"), "RobotDriveDevRef"=w186) -> ("error out"=w181:errorcluster, "RobotDriveDevRef"=w182:T11)  [unwired: 6 in, 1 out]
      n97 = call <vilib>:"WPI_RobotDriveDelayAndUpdateSafety.vi"("error in (no error)"=w181, "Delay (s)"=2.0, "RobotDriveDevRef"=w182) -> ("error out"=w178:errorcluster, "RobotDriveDevRef 2"=w179:T11)  [unwired: 7 in]
      n98 = call-poly <vilib>:"WPI_RobotDriveArcadeDrive.vi"("error in (no error)"=w178, "Y axis value"=0.0, "X axis value"=0.0, "RobotDriveDevRef"=w179) -> ()  [unwired: 5 in, 3 out]
    }
    frame "NEW" {
      n99 = while {
        tunnel: w263 -> [w355]
        tunnel: w262 -> [w354]
        tunnel: [w348] -> w264
        tunnel: [w347] -> w265
        tunnel: w261 -> [w346]
        tunnel: w260 -> [w340]
        tunnel: [w336] -> w259
        tunnel: [w335] -> w258
        tunnel: w249 -> [w334]
        tunnel: [w334] -> w248
        stop <- w337 stop-if-true
        n100 = call <vilib>:"WPI_EncoderGet.vi"("EncoderDevRef"=w346) -> ("Distance"=w345:dbl, "EncoderDevRef"=w336:T3)  [unwired: 5 in, 4 out]
        n101 = call <vilib>:"WPI_EncoderGet.vi"("EncoderDevRef"=w355) -> ("Distance"=w353:dbl, "EncoderDevRef"=w347:T3)  [unwired: 5 in, 4 out]
        n102 = Greater?(x=w345, y=4.0) -> (0:w338:bool)
        n103 = Greater?(x=w353, y=4.0) -> (0:w339:bool)
        n104 = Select(t=0.0, s=w338, f=-0.3) -> (s? t:f=w341:dbl)
        n105 = Select(t=0.0, s=w339, f=-0.3) -> (s? t:f=w349:dbl)
        n106 = And(x=w339, y=w338) -> (x .and. y?=w337:bool)
        n107 = call <vilib>:"WPI_MotorControlSetOutput.vi"("Output"=w341, "MotorControlDevRef"=w340) -> ("MotorControlDevRef"=w335:T7)  [unwired: 7 in, 2 out]
        n108 = call <vilib>:"WPI_MotorControlSetOutput.vi"("Output"=w349, "MotorControlDevRef"=w354) -> ("MotorControlDevRef"=w348:T7)  [unwired: 7 in, 2 out]
      }
      n109 = while {
        tunnel: [w330] -> w257
        tunnel: [w329] -> w256
        tunnel: w265 -> [w328]
        tunnel: w264 -> [w327]
        tunnel: w259 -> [w323]
        tunnel: w258 -> [w322]
        tunnel: [w323] -> w255
        tunnel: [w322] -> w254
        tunnel: w248 -> [w321]
        tunnel: [w321] -> w247
        stop <- w324 continue-if-true
        n110 = call <vilib>:"WPI_EncoderGet.vi"("EncoderDevRef"=w328) -> ("Distance"=w326:dbl, "EncoderDevRef"=w330:T3)  [unwired: 5 in, 4 out]
        n111 = Greater?(x=4.0 ("y"), y=w326) -> (0:w324:bool)
        n112 = Select(t=0.3, s=w324, f=0.0 ("Output")) -> (s? t:f=w331:dbl)
        n113 = call <vilib>:"WPI_MotorControlSetOutput.vi"("Output"=w331, "MotorControlDevRef"=w327) -> ("MotorControlDevRef"=w329:T7)  [unwired: 7 in, 2 out]
      }
      n114 = while {
        tunnel: w257 -> [w320]
        tunnel: w256 -> [w319]
        tunnel: [w313] -> w250
        tunnel: [w312] -> w251
        tunnel: w255 -> [w311]
        tunnel: w254 -> [w305]
        tunnel: [w301] -> w252
        tunnel: [w300] -> w253
        tunnel: w247 -> [w299]
        tunnel: [w299] -> w246
        stop <- w302 stop-if-true
        n115 = call <vilib>:"WPI_EncoderGet.vi"("EncoderDevRef"=w311) -> ("Distance"=w310:dbl, "EncoderDevRef"=w301:T3)  [unwired: 5 in, 4 out]
        n116 = call <vilib>:"WPI_EncoderGet.vi"("EncoderDevRef"=w320) -> ("Distance"=w318:dbl, "EncoderDevRef"=w312:T3)  [unwired: 5 in, 4 out]
        n117 = Greater?(x=w310, y=4.0) -> (0:w303:bool)
        n118 = Greater?(x=w318, y=4.0) -> (0:w304:bool)
        n119 = Select(t=0.0, s=w303, f=-0.3) -> (s? t:f=w306:dbl)
        n120 = Select(t=0.0, s=w304, f=-0.3) -> (s? t:f=w314:dbl)
        n121 = And(x=w304, y=w303) -> (x .and. y?=w302:bool)
        n122 = call <vilib>:"WPI_MotorControlSetOutput.vi"("Output"=w306, "MotorControlDevRef"=w305) -> ("MotorControlDevRef"=w300:T7)  [unwired: 7 in, 2 out]
        n123 = call <vilib>:"WPI_MotorControlSetOutput.vi"("Output"=w314, "MotorControlDevRef"=w319) -> ("MotorControlDevRef"=w313:T7)  [unwired: 7 in, 2 out]
      }
      n124 = while {
        tunnel: w253 -> [w290]
        tunnel: w252 -> [w289]
        tunnel: w251 -> [w287]
        tunnel: w250 -> [w288]
        tunnel: w246 -> [w298]
        tunnel: [w290] -> w245
        tunnel: [w289] -> w244
        tunnel: [w288] -> w243
        tunnel: [w287] -> w242
        stop <- w291 stop-if-true
        n125 = global read "Robot Global Data.vi" "LOWER LIMIT"() -> (w294:bool)
        n126 = Select(t=0.0, s=w294, f=-0.5) -> (s? t:f=w295:dbl)
        n127 = call <vilib>:"WPI_MotorControlSetOutput.vi"("Output"=w295, "MotorControlDevRef"=w298) -> ("Motor Output"=w293:dbl)  [unwired: 7 in, 2 out]
        n128 = Equal?(x=w293, y=0.0) -> (x = y?=w291:bool)
      }
      n129 = while {
        tunnel: [w281] -> _
        tunnel: [w280] -> _
        tunnel: [w271] -> _
        tunnel: [w270] -> _
        tunnel: w245 -> [w269]
        tunnel: w244 -> [w268]
        tunnel: w243 -> [w267]
        tunnel: w242 -> [w266]
        stop <- w272 stop-if-true
        n130 = call <vilib>:"WPI_EncoderGet.vi"("EncoderDevRef"=w268) -> ("Distance"=w279:dbl, "EncoderDevRef"=w271:T3)  [unwired: 5 in, 4 out]
        n131 = call <vilib>:"WPI_EncoderGet.vi"("EncoderDevRef"=w266) -> ("Distance"=w286:dbl, "EncoderDevRef"=w280:T3)  [unwired: 5 in, 4 out]
        n132 = Greater?(x=w279, y=0.0) -> (0:w273:bool)
        n133 = Greater?(x=w286, y=0.0) -> (0:w274:bool)
        n134 = Select(t=-0.3, s=w273, f=0.0) -> (s? t:f=w275:dbl)
        n135 = Select(t=-0.3, s=w274, f=0.0) -> (s? t:f=w282:dbl)
        n136 = And(x=w274, y=w273) -> (x .and. y?=w272:bool)
        n137 = call <vilib>:"WPI_MotorControlSetOutput.vi"("Output"=w275, "MotorControlDevRef"=w269) -> ("MotorControlDevRef"=w270:T7)  [unwired: 7 in, 2 out]
        n138 = call <vilib>:"WPI_MotorControlSetOutput.vi"("Output"=w282, "MotorControlDevRef"=w267) -> ("MotorControlDevRef"=w281:T7)  [unwired: 7 in, 2 out]
      }
    }
    frame "GEAR1" {
      n139 = while {
        tunnel: w374 -> [w455]
        tunnel: w375 -> [w435]
        tunnel: [w451] -> w370
        tunnel: [w450] -> w365
        tunnel: w373 -> [w442]
        tunnel: w372 -> [w439]
        tunnel: [w442] -> w363
        tunnel: [w446] -> w369
        tunnel: w371 -> [w445]
        tunnel: [w445] -> w367
        stop <- w440 continue-if-true
        n140 = call <vilib>:"WPI_CANTalonSRX_GetStatus.vi"("CAN Talon SRX Ref"=w435) -> ("Talon SRX Status"=w433:T15, "CAN Talon SRX Ref"=w434:T7)  [unwired: 8 in, 1 out]
        n141 = call <vilib>:"WPI_CANTalonSRX_GetStatus.vi"("CAN Talon SRX Ref"=w439) -> ("Talon SRX Status"=w437:T15, "CAN Talon SRX Ref"=w438:T7)  [unwired: 8 in, 1 out]
        n142 = Unbundle By Name(w437) -> ("Current"=→"CURRENT":dbl)
        n143 = call <vilib>:"WPI_EncoderGet.vi"("EncoderDevRef"=w455) -> ("Distance"=w441:dbl, "EncoderDevRef"=w450:T3)  [unwired: 5 in, 4 out]
        "Distance" <- w441
        n144 = Unbundle By Name(w433) -> ("Current"=→"Current":dbl)
        n145 = In Range and Coerce(upper limit=15.9, x=w441, lower limit=0.0) -> (In Range?=w440:bool)  [unwired: 1 out]
        n146 = Select(t=0.3, s=w440, f=0.0) -> (s? t:f=w447:dbl)
        n147 = Select(t=0.3, s=w440, f=0.0) -> (s? t:f=w452:dbl)
        n148 = call <vilib>:"WPI_MotorControlSetOutput.vi"("Output"=w447, "MotorControlDevRef"=w438) -> ("MotorControlDevRef"=w446:T7)  [unwired: 7 in, 2 out]
        n149 = call <vilib>:"WPI_MotorControlSetOutput.vi"("Output"=w452, "MotorControlDevRef"=w434) -> ("MotorControlDevRef"=w451:T7)  [unwired: 7 in, 2 out]
      }
      n150 = call <vilib>:"WPI_EncoderReset.vi"("EncoderDevRef"=w365) -> ("EncoderDevRef"=w364:T3)  [unwired: 9 in, 1 out]
      n151 = while {
        tunnel: [w411] -> w368
        tunnel: [w410] -> w362
        tunnel: [w406] -> w359
        tunnel: w364 -> [w402]
        tunnel: w370 -> [w401]
        tunnel: w369 -> [w400]
        tunnel: [w399] -> w366
        tunnel: w367 -> [w399]
        tunnel: w363 -> [w398]
        stop <- w392 continue-if-true
        n152 = call <vilib>:"WPI_EncoderGet.vi"("EncoderDevRef"=w398) -> ("Distance"=w397:dbl)  [unwired: 5 in, 5 out]
        n153 = call <vilib>:"WPI_EncoderGet.vi"("EncoderDevRef"=w402) -> ("Distance"=w403:dbl, "EncoderDevRef"=w410:T3)  [unwired: 5 in, 4 out]
        n154 = In Range and Coerce(upper limit=0.4, x=w397, lower limit=0.0) -> (In Range?=w394:bool)  [unwired: 1 out]
        n155 = In Range and Coerce(upper limit=5.9, x=w403, lower limit=0.0) -> (In Range?=w393:bool)  [unwired: 1 out]
        n156 = Select(t=0.3, s=w394, f=0.0) -> (s? t:f=w407:dbl)
        n157 = Select(t=-0.3, s=w393, f=0.0) -> (s? t:f=w412:dbl)
        n158 = And(x=w394, y=w393) -> (x .and. y?=w392:bool)
        n159 = call <vilib>:"WPI_MotorControlSetOutput.vi"("Output"=w407, "MotorControlDevRef"=w400) -> ("MotorControlDevRef"=w406:T7)  [unwired: 7 in, 2 out]
        n160 = call <vilib>:"WPI_MotorControlSetOutput.vi"("Output"=w412, "MotorControlDevRef"=w401) -> ("MotorControlDevRef"=w411:T7)  [unwired: 7 in, 2 out]
      }
      n161 = call <vilib>:"WPI_EncoderReset.vi"("EncoderDevRef"=w362) -> ("EncoderDevRef"=w361:T3)  [unwired: 9 in, 1 out]
      n162 = while {
        tunnel: [w428] -> w358
        tunnel: [w427] -> w357
        tunnel: [w423] -> w356
        tunnel: w368 -> [w418]
        tunnel: w359 -> [w417]
        tunnel: w366 -> [w415]
        tunnel: w361 -> [w416]
        tunnel: [w415] -> _
        stop <- w419 continue-if-true
        n163 = call <vilib>:"WPI_EncoderGet.vi"("EncoderDevRef"=w416) -> ("Distance"=w420:dbl, "EncoderDevRef"=w427:T3)  [unwired: 5 in, 4 out]
        n164 = In Range and Coerce(upper limit=5.0, x=w420, lower limit=0.0) -> (In Range?=w419:bool)  [unwired: 1 out]
        n165 = Select(t=-0.3, s=w419, f=0.0) -> (s? t:f=w424:dbl)
        n166 = Select(t=-0.3, s=w419, f=0.0) -> (s? t:f=w429:dbl)
        n167 = call <vilib>:"WPI_MotorControlSetOutput.vi"("Output"=w424, "MotorControlDevRef"=w417) -> ("MotorControlDevRef"=w423:T7)  [unwired: 7 in, 2 out]
        n168 = call <vilib>:"WPI_MotorControlSetOutput.vi"("Output"=w429, "MotorControlDevRef"=w418) -> ("MotorControlDevRef"=w428:T7)  [unwired: 7 in, 2 out]
      }
      n169 = call <vilib>:"WPI_EncoderReset.vi"("EncoderDevRef"=w357) -> ("EncoderDevRef"=w360:T3)  [unwired: 9 in, 1 out]
      n170 = while {
        tunnel: [w388] -> _
        tunnel: [w387] -> _
        tunnel: [w383] -> _
        tunnel: w358 -> [w378]
        tunnel: w356 -> [w377]
        tunnel: w360 -> [w376]
        stop <- w379 continue-if-true
        n171 = call <vilib>:"WPI_EncoderGet.vi"("EncoderDevRef"=w376) -> ("Distance"=w380:dbl, "EncoderDevRef"=w387:T3)  [unwired: 5 in, 4 out]
        n172 = In Range and Coerce(upper limit=5.0, x=w380, lower limit=0.0) -> (In Range?=w379:bool)  [unwired: 1 out]
        n173 = Select(t=0.4, s=w379, f=0.0) -> (s? t:f=w384:dbl)
        n174 = Select(t=0.4, s=w379, f=0.0) -> (s? t:f=w389:dbl)
        n175 = call <vilib>:"WPI_MotorControlSetOutput.vi"("Output"=w384, "MotorControlDevRef"=w377) -> ("MotorControlDevRef"=w383:T7)  [unwired: 7 in, 2 out]
        n176 = call <vilib>:"WPI_MotorControlSetOutput.vi"("Output"=w389, "MotorControlDevRef"=w378) -> ("MotorControlDevRef"=w388:T7)  [unwired: 7 in, 2 out]
      }
    }
    frame "ENCODER" {
      n177 = while {
        tunnel: w457 -> [w461]
        tunnel: w456 -> [w460]
        stop <- "stop" stop-if-true
        n178 = call <vilib>:"WPI_EncoderGet.vi"("EncoderDevRef"=w461) -> ("Distance"=→"PLAY 2":dbl)  [unwired: 5 in, 5 out]
        n179 = call <vilib>:"WPI_EncoderGet.vi"("EncoderDevRef"=w460) -> ("Distance"=→"PLAY 1":dbl)  [unwired: 5 in, 5 out]
      }
    }
    frame "AUTO CENTER" {
      n180 = while {
        tunnel: w476 -> [w531]
        tunnel: w475 -> [w530]
        tunnel: [w524] -> w467
        tunnel: [w523] -> w466
        tunnel: w474 -> [w522]
        tunnel: w473 -> [w516]
        tunnel: [w512] -> w465
        tunnel: [w511] -> w464
        tunnel: w472 -> [w510]
        tunnel: [w510] -> w463
        stop <- w513 stop-if-true
        n181 = call <vilib>:"WPI_EncoderGet.vi"("EncoderDevRef"=w522) -> ("Distance"=w521:dbl, "EncoderDevRef"=w512:T3)  [unwired: 5 in, 4 out]
        n182 = call <vilib>:"WPI_EncoderGet.vi"("EncoderDevRef"=w531) -> ("Distance"=w529:dbl, "EncoderDevRef"=w523:T3)  [unwired: 5 in, 4 out]
        n183 = Greater?(x=w521, y=4.0) -> (0:w514:bool)
        n184 = Greater?(x=w529, y=4.0) -> (0:w515:bool)
        n185 = Select(t=0.0, s=w514, f=-0.3) -> (s? t:f=w517:dbl)
        n186 = Select(t=0.0, s=w515, f=-0.3) -> (s? t:f=w525:dbl)
        n187 = And(x=w515, y=w514) -> (x .and. y?=w513:bool)
        n188 = call <vilib>:"WPI_MotorControlSetOutput.vi"("Output"=w517, "MotorControlDevRef"=w516) -> ("MotorControlDevRef"=w511:T7)  [unwired: 7 in, 2 out]
        n189 = call <vilib>:"WPI_MotorControlSetOutput.vi"("Output"=w525, "MotorControlDevRef"=w530) -> ("MotorControlDevRef"=w524:T7)  [unwired: 7 in, 2 out]
      }
      n190 = while {
        tunnel: w464 -> [w501]
        tunnel: w465 -> [w500]
        tunnel: w466 -> [w498]
        tunnel: w467 -> [w499]
        tunnel: w463 -> [w509]
        tunnel: [w501] -> w468
        tunnel: [w500] -> w469
        tunnel: [w499] -> w470
        tunnel: [w498] -> w471
        stop <- w502 stop-if-true
        n191 = global read "Robot Global Data.vi" "LOWER LIMIT"() -> (w505:bool)
        n192 = Select(t=0.0, s=w505, f=-0.5) -> (s? t:f=w506:dbl)
        n193 = call <vilib>:"WPI_MotorControlSetOutput.vi"("Output"=w506, "MotorControlDevRef"=w509) -> ("Motor Output"=w504:dbl)  [unwired: 7 in, 2 out]
        n194 = Equal?(x=w504, y=0.0) -> (x = y?=w502:bool)
      }
      n195 = while {
        tunnel: [w492] -> _
        tunnel: [w491] -> _
        tunnel: [w482] -> _
        tunnel: [w481] -> _
        tunnel: w468 -> [w480]
        tunnel: w469 -> [w479]
        tunnel: w470 -> [w478]
        tunnel: w471 -> [w477]
        stop <- w483 stop-if-true
        n196 = call <vilib>:"WPI_EncoderGet.vi"("EncoderDevRef"=w479) -> ("Distance"=w490:dbl, "EncoderDevRef"=w482:T3)  [unwired: 5 in, 4 out]
        n197 = call <vilib>:"WPI_EncoderGet.vi"("EncoderDevRef"=w477) -> ("Distance"=w497:dbl, "EncoderDevRef"=w491:T3)  [unwired: 5 in, 4 out]
        n198 = Greater?(x=w490, y=0.0) -> (0:w484:bool)
        n199 = Greater?(x=w497, y=0.0) -> (0:w485:bool)
        n200 = Select(t=-0.3, s=w484, f=0.0) -> (s? t:f=w486:dbl)
        n201 = Select(t=-0.3, s=w485, f=0.0) -> (s? t:f=w493:dbl)
        n202 = And(x=w485, y=w484) -> (x .and. y?=w483:bool)
        n203 = call <vilib>:"WPI_MotorControlSetOutput.vi"("Output"=w486, "MotorControlDevRef"=w480) -> ("MotorControlDevRef"=w481:T7)  [unwired: 7 in, 2 out]
        n204 = call <vilib>:"WPI_MotorControlSetOutput.vi"("Output"=w493, "MotorControlDevRef"=w478) -> ("MotorControlDevRef"=w492:T7)  [unwired: 7 in, 2 out]
      }
    }
    frame "AUTO LEFT NS" {
      n205 = while {
        tunnel: w551 -> [w605]
        tunnel: w550 -> [w604]
        tunnel: [w600] -> w545
        tunnel: [w599] -> w546
        tunnel: w549 -> [w590]
        tunnel: w548 -> [w595]
        tunnel: [w590] -> w544
        tunnel: [w594] -> w543
        tunnel: w547 -> [w593]
        tunnel: [w593] -> w542
        stop <- w588 continue-if-true
        n206 = call <vilib>:"WPI_EncoderGet.vi"("EncoderDevRef"=w605) -> ("Distance"=w589:dbl, "EncoderDevRef"=w599:T3)  [unwired: 5 in, 4 out]
        "Distance 3" <- w589
        n207 = In Range and Coerce(upper limit=12.0, x=w589, lower limit=0.0) -> (In Range?=w588:bool)  [unwired: 1 out]
        n208 = Select(t=0.35, s=w588, f=0.0) -> (s? t:f=w596:dbl)
        n209 = Select(t=0.35, s=w588, f=0.0) -> (s? t:f=w601:dbl)
        n210 = call <vilib>:"WPI_MotorControlSetOutput.vi"("Output"=w596, "MotorControlDevRef"=w595) -> ("MotorControlDevRef"=w594:T7)  [unwired: 7 in, 2 out]
        n211 = call <vilib>:"WPI_MotorControlSetOutput.vi"("Output"=w601, "MotorControlDevRef"=w604) -> ("MotorControlDevRef"=w600:T7)  [unwired: 7 in, 2 out]
      }
      n212 = while {
        tunnel: w546 -> [w587]
        tunnel: w545 -> [w586]
        tunnel: [w582] -> w540
        tunnel: [w581] -> w541
        tunnel: w544 -> [w572]
        tunnel: w543 -> [w577]
        tunnel: [w572] -> w539
        tunnel: [w576] -> w538
        tunnel: w542 -> [w575]
        tunnel: [w575] -> w537
        stop <- w570 continue-if-true
        n213 = call <vilib>:"WPI_EncoderGet.vi"("EncoderDevRef"=w587) -> ("Distance"=w571:dbl, "EncoderDevRef"=w581:T3)  [unwired: 5 in, 4 out]
        "Distance 4" <- w571
        n214 = In Range and Coerce(upper limit=2.4, x=w571, lower limit=0.0) -> (In Range?=w570:bool)  [unwired: 1 out]
        n215 = Select(t=0.0, s=w570, f=0.0) -> (s? t:f=w578:dbl)
        n216 = Select(t=0.35, s=w570, f=0.0) -> (s? t:f=w583:dbl)
        n217 = call <vilib>:"WPI_MotorControlSetOutput.vi"("Output"=w578, "MotorControlDevRef"=w577) -> ("MotorControlDevRef"=w576:T7)  [unwired: 7 in, 2 out]
        n218 = call <vilib>:"WPI_MotorControlSetOutput.vi"("Output"=w583, "MotorControlDevRef"=w586) -> ("MotorControlDevRef"=w582:T7)  [unwired: 7 in, 2 out]
      }
      n219 = while {
        tunnel: w541 -> [w569]
        tunnel: w540 -> [w568]
        tunnel: [w564] -> w536
        tunnel: [w563] -> w535
        tunnel: w539 -> [w554]
        tunnel: w538 -> [w559]
        tunnel: [w554] -> w534
        tunnel: [w558] -> w533
        tunnel: w537 -> [w557]
        tunnel: [w557] -> w532
        stop <- w552 continue-if-true
        n220 = call <vilib>:"WPI_EncoderGet.vi"("EncoderDevRef"=w569) -> ("Distance"=w553:dbl, "EncoderDevRef"=w563:T3)  [unwired: 5 in, 4 out]
        "Distance 5" <- w553
        n221 = In Range and Coerce(upper limit=4.0, x=w553, lower limit=0.0) -> (In Range?=w552:bool)  [unwired: 1 out]
        n222 = Select(t=0.35, s=w552, f=0.0) -> (s? t:f=w560:dbl)
        n223 = Select(t=0.35, s=w552, f=0.0) -> (s? t:f=w565:dbl)
        n224 = call <vilib>:"WPI_MotorControlSetOutput.vi"("Output"=w560, "MotorControlDevRef"=w559) -> ("MotorControlDevRef"=w558:T7)  [unwired: 7 in, 2 out]
        n225 = call <vilib>:"WPI_MotorControlSetOutput.vi"("Output"=w565, "MotorControlDevRef"=w568) -> ("MotorControlDevRef"=w564:T7)  [unwired: 7 in, 2 out]
      }
      n226 = while {
        tunnel: w533 -> [w610]
        tunnel: w534 -> [w609]
        tunnel: w535 -> [w607]
        tunnel: w536 -> [w608]
        tunnel: w532 -> [w618]
        tunnel: [w610] -> _
        tunnel: [w609] -> _
        tunnel: [w608] -> _
        tunnel: [w607] -> _
        tunnel: [w606] -> _
        stop <- w611 stop-if-true
        n227 = global read "Robot Global Data.vi" "LOWER LIMIT"() -> (w614:bool)
        n228 = Select(t=0.0, s=w614, f=-0.5) -> (s? t:f=w615:dbl)
        n229 = call <vilib>:"WPI_MotorControlSetOutput.vi"("Output"=w615, "MotorControlDevRef"=w618) -> ("Motor Output"=w613:dbl, "MotorControlDevRef"=w606:T7)  [unwired: 7 in, 1 out]
        n230 = Equal?(x=w613, y=0.0) -> (x = y?=w611:bool)
      }
    }
    frame "MIDDLE" {
      n231 = call-poly <vilib>:"WPI_RobotDriveArcadeDrive.vi"("error in (no error)"=w648, "Y axis value"=0.45, "RobotDriveDevRef"=w649) -> ("error out"=w645:errorcluster, "RobotDriveDevRef"=w646:T11)  [unwired: 6 in, 1 out]
      n232 = call <vilib>:"WPI_RobotDriveDelayAndUpdateSafety.vi"("error in (no error)"=w645, "Delay (s)"=2.0, "RobotDriveDevRef"=w646) -> ("error out"=w643:errorcluster, "RobotDriveDevRef 2"=w642:T11)  [unwired: 7 in]
      n233 = call-poly <vilib>:"WPI_RobotDriveArcadeDrive.vi"("error in (no error)"=w643, "Y axis value"=0.0, "RobotDriveDevRef"=w642) -> ("error out"=w639:errorcluster, "RobotDriveDevRef"=w640:T11)  [unwired: 6 in, 1 out]
      n234 = call <vilib>:"WPI_RobotDriveDelayAndUpdateSafety.vi"("error in (no error)"=w639, "Delay (s)"=0.5, "RobotDriveDevRef"=w640) -> ("error out"=w637:errorcluster, "RobotDriveDevRef 2"=w635:T11)  [unwired: 7 in]
      n235 = call <vilib>:"WPI_MotorControlSetOutput.vi"("error in (no error)"=w637, "Output"=-0.7, "MotorControlDevRef"=w636) -> ("error out"=w634:errorcluster, "MotorControlDevRef"=w630:T7)  [unwired: 6 in, 1 out]
      n236 = call <vilib>:"WPI_RobotDriveDelayAndUpdateSafety.vi"("error in (no error)"=w634, "Delay (s)"=1.5, "RobotDriveDevRef"=w635) -> ("error out"=w631:errorcluster, "RobotDriveDevRef 2"=w628:T11)  [unwired: 7 in]
      n237 = call <vilib>:"WPI_MotorControlSetOutput.vi"("error in (no error)"=w631, "Output"=0.0, "MotorControlDevRef"=w630) -> ("error out"=w627:errorcluster)  [unwired: 6 in, 2 out]
      n238 = call-poly <vilib>:"WPI_RobotDriveArcadeDrive.vi"("error in (no error)"=w627, "Y axis value"=-0.4, "RobotDriveDevRef"=w628) -> ("error out"=w624:errorcluster, "RobotDriveDevRef"=w625:T11)  [unwired: 6 in, 1 out]
      n239 = call <vilib>:"WPI_RobotDriveDelayAndUpdateSafety.vi"("error in (no error)"=w624, "Delay (s)"=2.0, "RobotDriveDevRef"=w625) -> ("error out"=w621:errorcluster, "RobotDriveDevRef 2"=w622:T11)  [unwired: 7 in]
      n240 = call-poly <vilib>:"WPI_RobotDriveArcadeDrive.vi"("error in (no error)"=w621, "Y axis value"=0.0, "X axis value"=0.0, "RobotDriveDevRef"=w622) -> ()  [unwired: 5 in, 3 out]
    }
    frame "RIGHTSIDE" {
      # "RIGHTSIDE"
      n241 = call-poly <vilib>:"WPI_RobotDriveArcadeDrive.vi"("error in (no error)"=w651, "Y axis value"=0.59, "RobotDriveDevRef"=w652) -> ("error out"=w691:errorcluster, "RobotDriveDevRef"=w692:T11)  [unwired: 6 in, 1 out]
      n242 = call <vilib>:"WPI_RobotDriveDelayAndUpdateSafety.vi"("error in (no error)"=w691, "Delay (s)"=1.8, "RobotDriveDevRef"=w692) -> ("error out"=w687:errorcluster, "RobotDriveDevRef 2"=w688:T11)  [unwired: 7 in]
      n243 = call-poly <vilib>:"WPI_RobotDriveArcadeDrive.vi"("error in (no error)"=w687, "X axis value"=0.36, "RobotDriveDevRef"=w688) -> ("error out"=w684:errorcluster, "RobotDriveDevRef"=w685:T11)  [unwired: 6 in, 1 out]
      n244 = call <vilib>:"WPI_RobotDriveDelayAndUpdateSafety.vi"("error in (no error)"=w684, "Delay (s)"=1.0, "RobotDriveDevRef"=w685) -> ("error out"=w681:errorcluster, "RobotDriveDevRef 2"=w682:T11)  [unwired: 7 in]
      n245 = call-poly <vilib>:"WPI_RobotDriveArcadeDrive.vi"("error in (no error)"=w681, "Y axis value"=0.5, "RobotDriveDevRef"=w682) -> ("error out"=w678:errorcluster, "RobotDriveDevRef"=w679:T11)  [unwired: 6 in, 1 out]
      n246 = call <vilib>:"WPI_RobotDriveDelayAndUpdateSafety.vi"("error in (no error)"=w678, "Delay (s)"=2.3, "RobotDriveDevRef"=w679) -> ("error out"=w675:errorcluster, "RobotDriveDevRef 2"=w676:T11)  [unwired: 7 in]
      n247 = call-poly <vilib>:"WPI_RobotDriveArcadeDrive.vi"("error in (no error)"=w675, "Y axis value"=0.0, "RobotDriveDevRef"=w676) -> ("error out"=w672:errorcluster, "RobotDriveDevRef"=w673:T11)  [unwired: 6 in, 1 out]
      n248 = call <vilib>:"WPI_RobotDriveDelayAndUpdateSafety.vi"("error in (no error)"=w672, "Delay (s)"=0.5, "RobotDriveDevRef"=w673) -> ("error out"=w670:errorcluster, "RobotDriveDevRef 2"=w668:T11)  [unwired: 7 in]
      n249 = call <vilib>:"WPI_MotorControlSetOutput.vi"("error in (no error)"=w670, "Output"=-0.7, "MotorControlDevRef"=w650) -> ("error out"=w667:errorcluster, "MotorControlDevRef"=w656:T7)  [unwired: 6 in, 1 out]
      n250 = call <vilib>:"WPI_RobotDriveDelayAndUpdateSafety.vi"("error in (no error)"=w667, "Delay (s)"=1.5, "RobotDriveDevRef"=w668) -> ("error out"=w655:errorcluster, "RobotDriveDevRef 2"=w665:T11)  [unwired: 7 in]
      n251 = call <vilib>:"WPI_MotorControlSetOutput.vi"("error in (no error)"=w655, "Output"=0.0, "MotorControlDevRef"=w656) -> ("error out"=w653:errorcluster)  [unwired: 6 in, 2 out]
      n252 = call-poly <vilib>:"WPI_RobotDriveArcadeDrive.vi"("error in (no error)"=w653, "Y axis value"=-0.4, "RobotDriveDevRef"=w665) -> ("error out"=w662:errorcluster, "RobotDriveDevRef"=w663:T11)  [unwired: 6 in, 1 out]
      n253 = call <vilib>:"WPI_RobotDriveDelayAndUpdateSafety.vi"("error in (no error)"=w662, "Delay (s)"=2.0, "RobotDriveDevRef"=w663) -> ("error out"=w660:errorcluster, "RobotDriveDevRef 2"=w659:T11)  [unwired: 7 in]
      n254 = call-poly <vilib>:"WPI_RobotDriveArcadeDrive.vi"("error in (no error)"=w660, "Y axis value"=0.0, "X axis value"=0.0, "RobotDriveDevRef"=w659) -> ()  [unwired: 5 in, 3 out]
    }
    frame "LEFTSIDE" {
      n255 = call-poly <vilib>:"WPI_RobotDriveArcadeDrive.vi"("error in (no error)"=w734, "Y axis value"=0.6, "RobotDriveDevRef"=w735) -> ("error out"=w732:errorcluster, "RobotDriveDevRef"=w733:T11)  [unwired: 6 in, 1 out]
      n256 = call <vilib>:"WPI_RobotDriveDelayAndUpdateSafety.vi"("error in (no error)"=w732, "Delay (s)"=2.0, "RobotDriveDevRef"=w733) -> ("error out"=w728:errorcluster, "RobotDriveDevRef 2"=w729:T11)  [unwired: 7 in]
      n257 = call-poly <vilib>:"WPI_RobotDriveArcadeDrive.vi"("error in (no error)"=w728, "X axis value"=-0.45, "RobotDriveDevRef"=w729) -> ("error out"=w725:errorcluster, "RobotDriveDevRef"=w726:T11)  [unwired: 6 in, 1 out]
      n258 = call <vilib>:"WPI_RobotDriveDelayAndUpdateSafety.vi"("error in (no error)"=w725, "Delay (s)"=1.0, "RobotDriveDevRef"=w726) -> ("error out"=w722:errorcluster, "RobotDriveDevRef 2"=w723:T11)  [unwired: 7 in]
      n259 = call-poly <vilib>:"WPI_RobotDriveArcadeDrive.vi"("error in (no error)"=w722, "Y axis value"=0.52, "RobotDriveDevRef"=w723) -> ("error out"=w719:errorcluster, "RobotDriveDevRef"=w720:T11)  [unwired: 6 in, 1 out]
      n260 = call <vilib>:"WPI_RobotDriveDelayAndUpdateSafety.vi"("error in (no error)"=w719, "Delay (s)"=2.25, "RobotDriveDevRef"=w720) -> ("error out"=w716:errorcluster, "RobotDriveDevRef 2"=w717:T11)  [unwired: 7 in]
      n261 = call-poly <vilib>:"WPI_RobotDriveArcadeDrive.vi"("error in (no error)"=w716, "Y axis value"=0.0, "RobotDriveDevRef"=w717) -> ("error out"=w713:errorcluster, "RobotDriveDevRef"=w714:T11)  [unwired: 6 in, 1 out]
      n262 = call <vilib>:"WPI_RobotDriveDelayAndUpdateSafety.vi"("error in (no error)"=w713, "Delay (s)"=0.5, "RobotDriveDevRef"=w714) -> ("error out"=w710:errorcluster, "RobotDriveDevRef 2"=w708:T11)  [unwired: 7 in]
      n263 = call <vilib>:"WPI_MotorControlSetOutput.vi"("error in (no error)"=w710, "Output"=-0.7, "MotorControlDevRef"=w711) -> ("error out"=w707:errorcluster, "MotorControlDevRef"=w696:T7)  [unwired: 6 in, 1 out]
      n264 = call <vilib>:"WPI_RobotDriveDelayAndUpdateSafety.vi"("error in (no error)"=w707, "Delay (s)"=1.5, "RobotDriveDevRef"=w708) -> ("error out"=w695:errorcluster, "RobotDriveDevRef 2"=w705:T11)  [unwired: 7 in]
      n265 = call <vilib>:"WPI_MotorControlSetOutput.vi"("error in (no error)"=w695, "Output"=0.0, "MotorControlDevRef"=w696) -> ("error out"=w693:errorcluster)  [unwired: 6 in, 2 out]
      n266 = call-poly <vilib>:"WPI_RobotDriveArcadeDrive.vi"("error in (no error)"=w693, "Y axis value"=-0.4, "RobotDriveDevRef"=w705) -> ("error out"=w702:errorcluster, "RobotDriveDevRef"=w703:T11)  [unwired: 6 in, 1 out]
      n267 = call <vilib>:"WPI_RobotDriveDelayAndUpdateSafety.vi"("error in (no error)"=w702, "Delay (s)"=2.0, "RobotDriveDevRef"=w703) -> ("error out"=w700:errorcluster, "RobotDriveDevRef 2"=w699:T11)  [unwired: 7 in]
      n268 = call-poly <vilib>:"WPI_RobotDriveArcadeDrive.vi"("error in (no error)"=w700, "Y axis value"=0.0, "X axis value"=0.0, "RobotDriveDevRef"=w699) -> ()  [unwired: 5 in, 3 out]
    }
    frame "Forward" {
      n269 = call-poly <vilib>:"WPI_RobotDriveArcadeDrive.vi"("error in (no error)"=w740, "Y axis value"=0.55, "RobotDriveDevRef"=w741) -> ("error out"=w736:errorcluster, "RobotDriveDevRef"=w738:T11)  [unwired: 6 in, 1 out]
      n270 = call <vilib>:"WPI_RobotDriveDelayAndUpdateSafety.vi"("error in (no error)"=w736, "Delay (s)"=2.8, "RobotDriveDevRef"=w738) -> ()  [unwired: 7 in, 2 out]
    }
    frame "GEAR DROP" {
      n271 = call-poly <vilib>:"WPI_RobotDriveArcadeDrive.vi"("error in (no error)"=w765, "Y axis value"=0.45, "RobotDriveDevRef"=w766) -> ("error out"=w762:errorcluster, "RobotDriveDevRef"=w763:T11)  [unwired: 6 in, 1 out]
      n272 = call <vilib>:"WPI_RobotDriveDelayAndUpdateSafety.vi"("error in (no error)"=w762, "Delay (s)"=2.4, "RobotDriveDevRef"=w763) -> ("error out"=w760:errorcluster, "RobotDriveDevRef 2"=w759:T11)  [unwired: 7 in]
      n273 = call-poly <vilib>:"WPI_RobotDriveArcadeDrive.vi"("error in (no error)"=w760, "Y axis value"=0.0, "RobotDriveDevRef"=w759) -> ("error out"=w756:errorcluster, "RobotDriveDevRef"=w757:T11)  [unwired: 6 in, 1 out]
      n274 = call <vilib>:"WPI_RobotDriveDelayAndUpdateSafety.vi"("error in (no error)"=w756, "Delay (s)"=0.5, "RobotDriveDevRef"=w757) -> ("error out"=w749:errorcluster, "RobotDriveDevRef 2"=w748:T11)  [unwired: 7 in]
      n275 = while {
        tunnel: w749 -> [w778]
        tunnel: [w775] -> w747
        tunnel: w746 -> [w774]
        tunnel: [w773] -> w745
        stop <- w776 stop-if-true
        n276 = global read "Robot Global Data.vi" "LOWER LIMIT"() -> (w776:bool)
        n277 = call <vilib>:"WPI_MotorControlSetOutput.vi"("error in (no error)"=w778, "Output"=-0.6 ("f"), "MotorControlDevRef"=w774) -> ("error out"=w775:errorcluster, "MotorControlDevRef"=w773:T7)  [unwired: 6 in, 1 out]
      }
      n278 = call-poly <vilib>:"WPI_RobotDriveArcadeDrive.vi"("error in (no error)"=w747, "Y axis value"=-0.4, "RobotDriveDevRef"=w748) -> ("error out"=w753:errorcluster, "RobotDriveDevRef"=w752:T11)  [unwired: 6 in, 1 out]
      n279 = call <vilib>:"WPI_RobotDriveDelayAndUpdateSafety.vi"("error in (no error)"=w753, "Delay (s)"=1.5, "RobotDriveDevRef"=w752) -> ("error out"=w744:errorcluster)  [unwired: 7 in, 1 out]
      n280 = while {
        tunnel: w745 -> [w771]
        tunnel: w744 -> [w769]
        tunnel: [w768] -> w743
        tunnel: [w767] -> w742
        stop <- w772 stop-if-true
        n281 = call <vilib>:"WPI_MotorControlSetOutput.vi"("error in (no error)"=w769, "Output"=0.6, "MotorControlDevRef"=w771) -> ("error out"=w767:errorcluster, "MotorControlDevRef"=w768:T7)  [unwired: 6 in, 1 out]
        n282 = global read "Robot Global Data.vi" "UPPER LIMIT"() -> (w772:bool)
      }
      n283 = call <vilib>:"WPI_MotorControlSetOutput.vi"("error in (no error)"=w742, "Output"=0.0, "MotorControlDevRef"=w743) -> ()  [unwired: 6 in, 3 out]
    }
  }
